vi "Interface_ImplementInterface.vi"(7 "Action":T1=enum."GeneratePattern", 8 "error in (no error)":errorcluster, 10 "DataIn":variant, 11 "ClassRefToActOn":refnum<vi>) -> (0 "error out":errorcluster, 1 "Name":string, 2 "DataOut":variant, 3 "Cancelled":bool)   [LabVIEW 2012]
uses:
  <resource>/Framework/Providers/Open_GDS/ClassProviders/Provider_BaseClassInterface/BaseProvider_SubVIs/BaseProvider_DesignPatternsActions.ctl
  <resource>/Framework/Providers/Open_GDS/ClassProviders/DesignPatterns/Interface/Interface_SubVIs/InterfaceType.ctl
  <resource>/Framework/Providers/Open_GDS/ClassProviders/Common/LvIcon_class/GDSLvIcon_ClassColorTypes.ctl
  <vilib>/picture/picture.llb/imagedata.ctl
  <vilib>/Utility/miscctls.llb/LVPointTypeDef.ctl
  <resource>/Framework/Providers/Open_GDS/ClassProviders/Provider_BaseClassInterface/ClassWriter_class/ClassWriter.lvclass
panel:
  in  "Interfaces":u16(ring) items=["I1-GOOP4.lvclass (By VI Server)", "I1-Native.lvclass (By VI Server)"]
  in  "_Cancel":bool
  in  "_OK":bool
  # "Implement Interface"
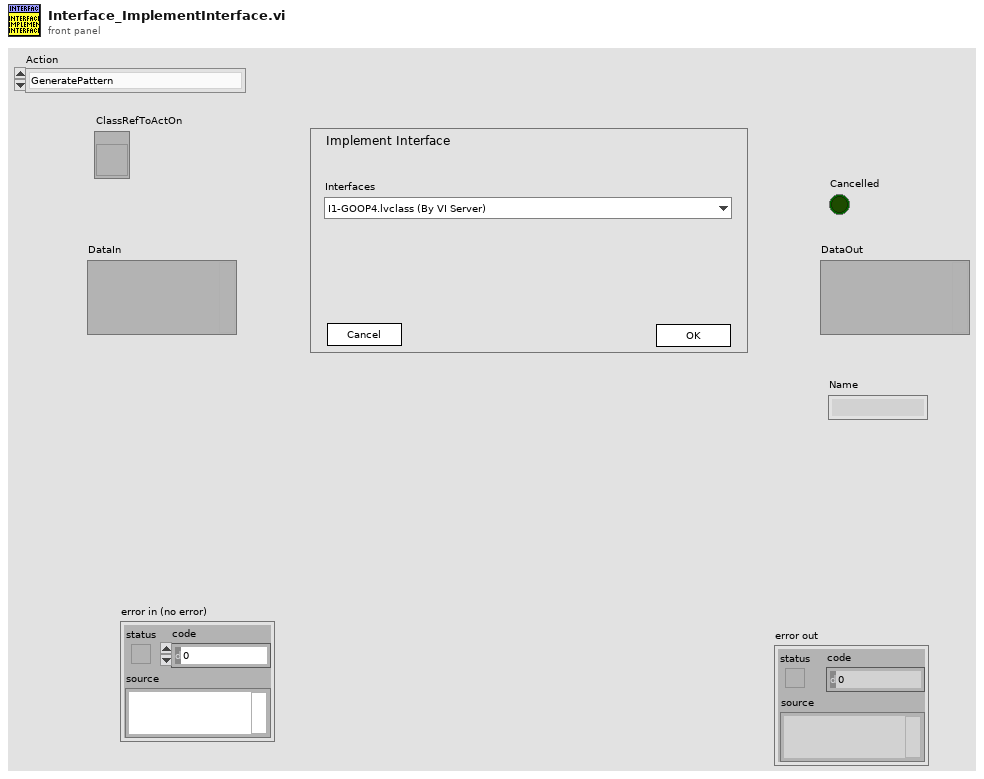
[diagram p1: front panel]
types:
  T1 = typedef "BaseProvider_DesignPatternsActions.ctl" = enum16{"AddPatternDialog", "GeneratePattern", "RemovePattern", "CreatePatternMethod", "UpdatePattern"}
  T2 = typedef "InterfaceType.ctl" = enum16{"ByAggregation", "ByViServer"}
  T3 = cluster{"Application":refnum<vi>, "ClassName":string, "BaseInterfaceClass":path, "ClassFolder":path, "BaseInterfaceClassRef":refnum<vi>, "NewInterfaceClassRef":refnum<vi>, "I_MethodRefs":refnum<vi>[], "C_MethodRefs":refnum<vi>[], "SubViUpperLeftTerminal":refnum<vi>[], "RefNameInSubInterface":string, "GetRefVI":path, "BaseInterfaceName":string, "RefNameInClass":string, "ImplementVI":path, "SubInterfaceImplementVI":path, "GetVIRef":refnum<vi>, "ImplementViRef":refnum<vi>, "SubInterfaceClassName":string, "FullClassName":string, "Type":T2}
  T4 = enum32{"Invalid", "Default", "Floating", "Floating/Auto-Hide", "Modal"}
  T5 = cluster{"Cancelled":bool, "Files":path[], "ClassPath":path, "DataOut":variant, "Interfaces":refnum<vi>[], "Type":T2[]}
  T6 = typedef "GDSLvIcon_ClassColorTypes.ctl" = cluster{"Frame":u32, "Header Text Color":u32, "Header Background":u32, "BodyBackgroundPublic":u32, "BodyBackgroundProtected":u32, "BodyBackgroundPrivate":u32, "Body Text Color":u32, "Frame thickness":u8, "ProtectedPrivateSame":bool, "Icon Header Size":u8, "Font Compression":enum16{"Auto", "On", "Off"}, "CapitalOnly":bool}
  T7 = typedef "imagedata.ctl" = cluster{"image type":i32, "image depth":i32, "image":u8[], "mask":u8[], "colors":u32[], "Rectangle":cluster{"left":i16, "top":i16, "right":i16, "bottom":i16}}
  T8 = enum16{"UINT8", "INT8", "UINT16", "INT16", "UINT32", "INT32", "UINT64", "INT64", "SGL", "DBL", "EXT", "CSG", "CDB", "CXT", "TimeStamp", "STRING", "PATH", "BOOL", "ENUM", "RefNum", "VIRefNum", "ClassRefNum", "Cluster", "Variant", "TypeRef", "Waveform", "LabVIEW Object", "Other"}
  T9 = typedef "LVPointTypeDef.ctl" = cluster{"Horizontal":i16, "Vertical":i16}
  T10 = typedef "GDSLvCLass_ClassSettingsType.ctl" = cluster{"ClassProviderName":string, "ClassTemplateUsed":string, "ClassTemplateVersion":string, "ClassDescription":string, "PlugIns":T11[], "ConnectorPanePattern":string}
  T11 = typedef "GDSLvClass_PlugIn.ctl" = cluster{"Type":T12, "ID":string, "Version":string, "Path":path, "Name":string, "Data":variant}
  T12 = typedef "GDSLvClass_PlugInTypes.ctl" = enum16{"DesignPattern", "MethodTypes"}
  T13 = typedef "GDSLvClass_IconSettingsType.ctl" = cluster{"Frame":u32, "Frame thickness":u8, "Header Background":u32, "Header Text":u32, "ColorPublic":u32, "ColorProtected":u32, "ColorPrivate":u32, "Body Text":u32, "ClassBodyIcon":string}
  T14 = cluster{"Foreground Color":u32, "Background Color":u32, "Fill Pattern":cluster{"Row 0":u8, "Row 1":u8, "Row 2":u8, "Row 3":u8, "Row 4":u8, "Row 5":u8, "Row 6":u8, "Row 7":u8}, "Width":i16, "Mode":enum16{"Copy", "Or", "Exclusive Or", "Bit Clear", "Not Copy", "Not Or", "Nor Exclusive Or", "Not Bit Clear"}, "Style":enum32{"Solid", "Dash", "Dot", "Dash Dot", "Dash Dot Dot"}, "Fill Rule":enum32{"Even Odd", "Winding"}, "End Caps":enum32{"Default", "Flat"}}[]
  T15 = enum16{"UINT8", "INT8", "UINT16", "INT16", "UINT32", "INT32", "UINT64", "INT64", "SGL", "DBL", "EXT", "CSG", "CDB", "CXT", "TimeStamp", "STRING", "PATH", "BOOL", "ENUM", "RefNum", "VIRefNum", "ClassRefNum", "Cluster", "Variant", "TypeRef", "Waveform", "LabVIEW Object", "Other"}[]
  T16 = typedef "LVRectTypeDef.ctl" = cluster{"Left":i16, "Top":i16, "Right":i16, "Bottom":i16}
  T17 = typedef "LVPositionTypeDef.ctl" = cluster{"Left":i32, "Top":i32}
  T18 = cluster{"Alignment":enum32{"Left", "Right", "Hybrid", "Center", "Gravity"}, "Rules":enum32{"Strict", "Allow Wires Under Labels", "Allow Wires Under Lead Nodes", "Allow Wires Under Wide Blocks"}, "Max Heuristic Iterations":u32, "Max Simplex Iterations":u32, "Block Padding":cluster{"Horizontal":i32, "Vertical":i32}, "Wire Padding":cluster{"Horizontal":i32, "Vertical":i32}, "Auto-Tune by Topology":bool, "Fine-Tune Y Positions":bool, "Align All Controls on Left":bool, "Align All Indicators on Right":bool, "Use Array Dimension Heuristics":bool}
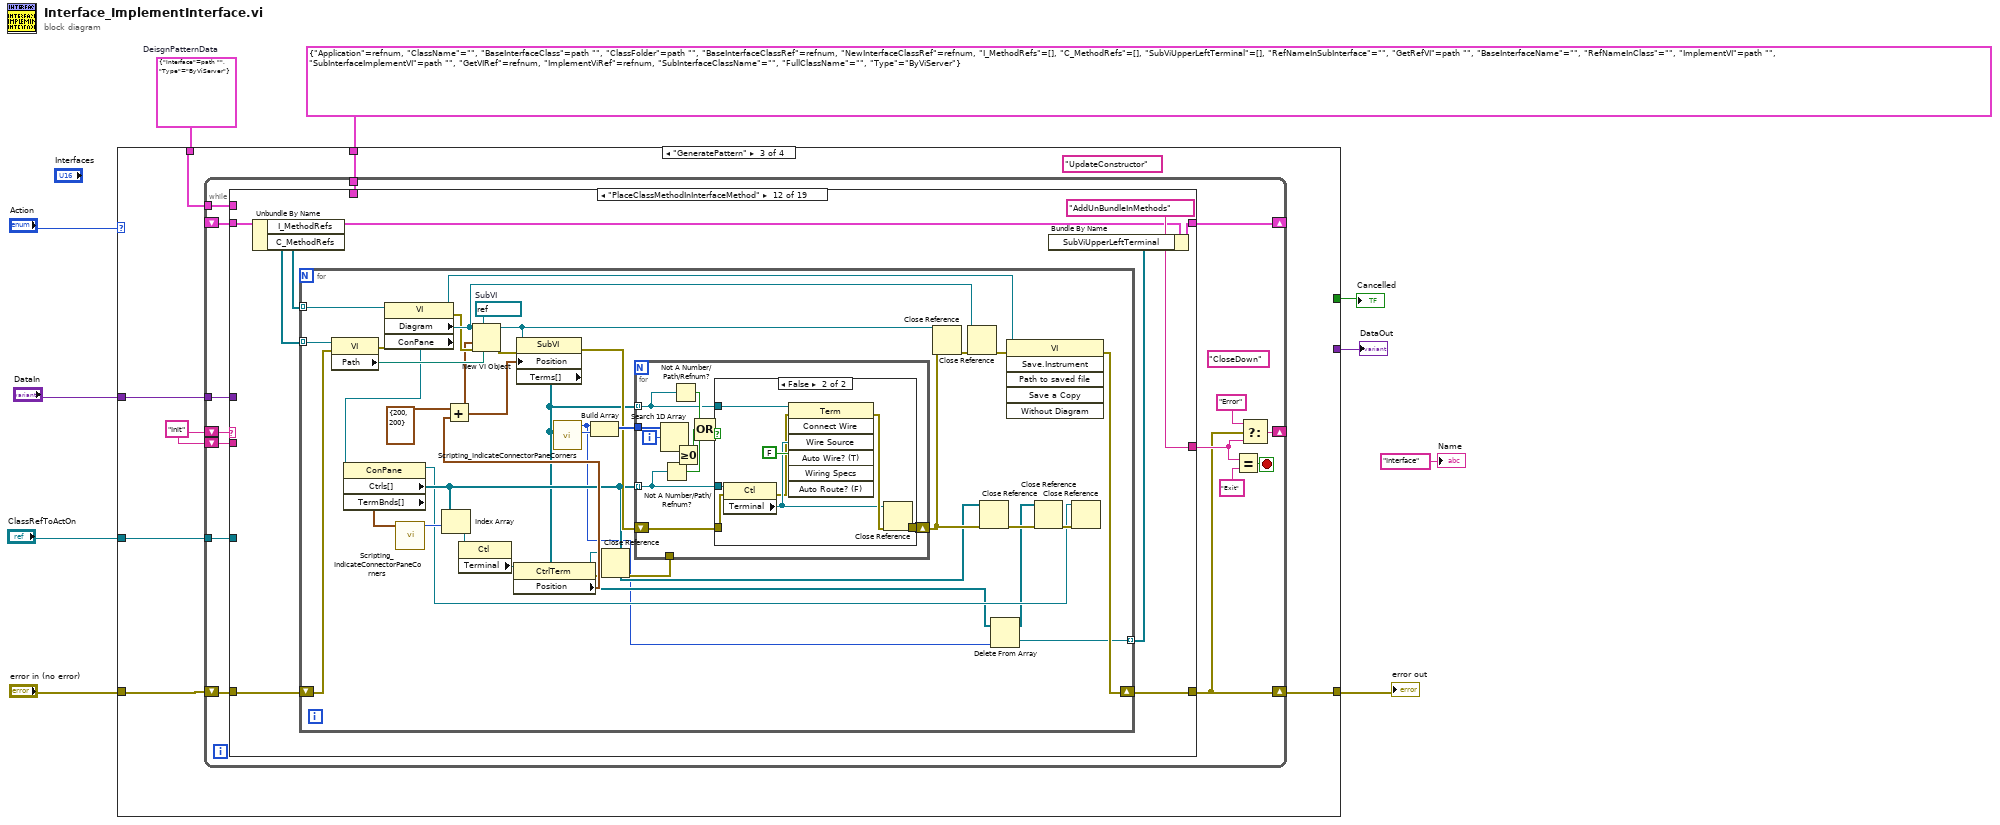
[diagram p0: block diagram]
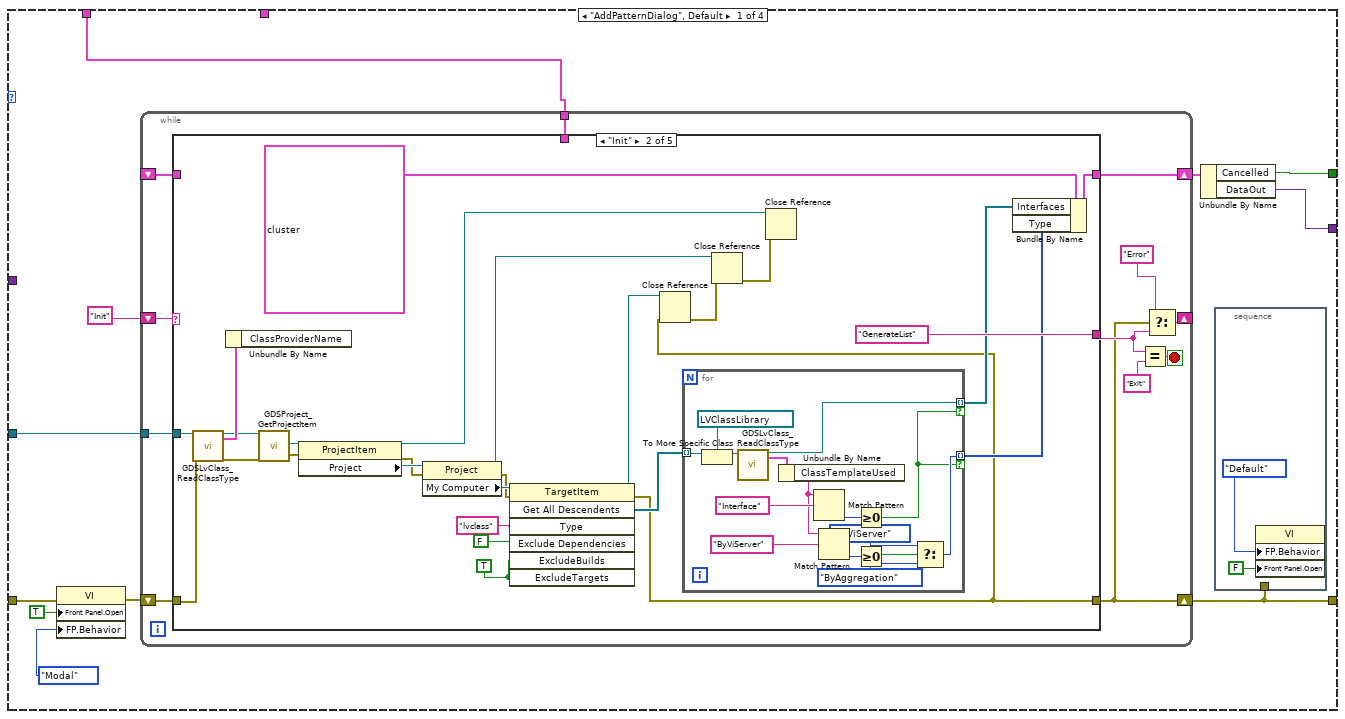
[diagram p2: hidden frame]
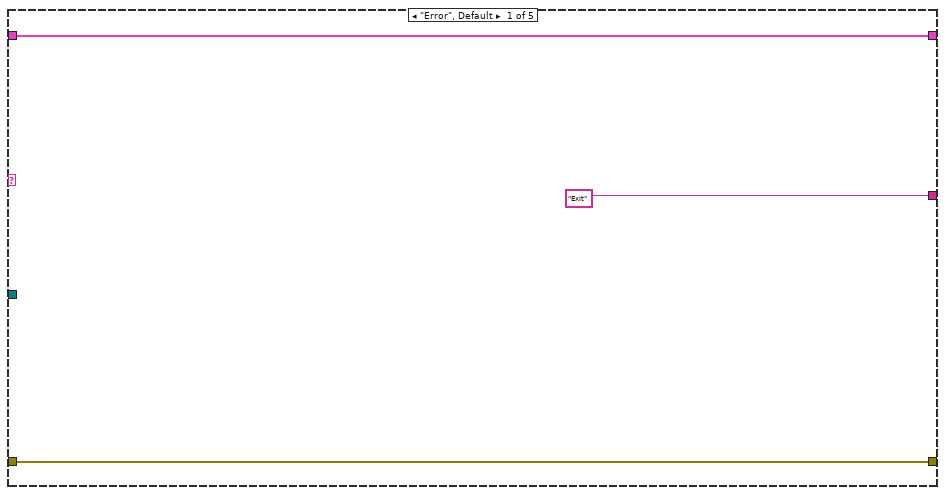
[diagram p3: hidden frame]
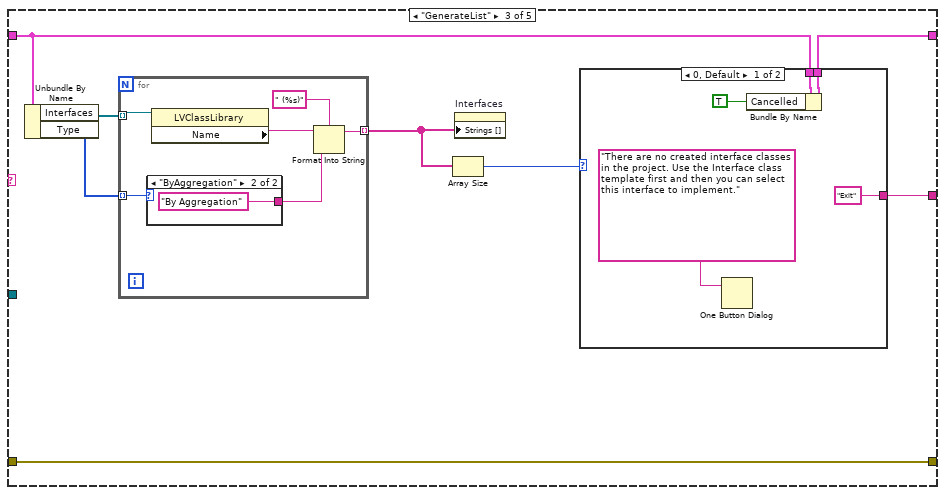
[diagram p4: hidden frame]
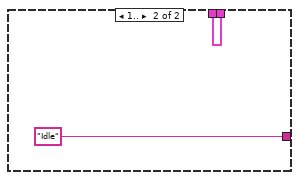
[diagram p5: hidden frame]
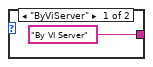
[diagram p6: hidden frame]
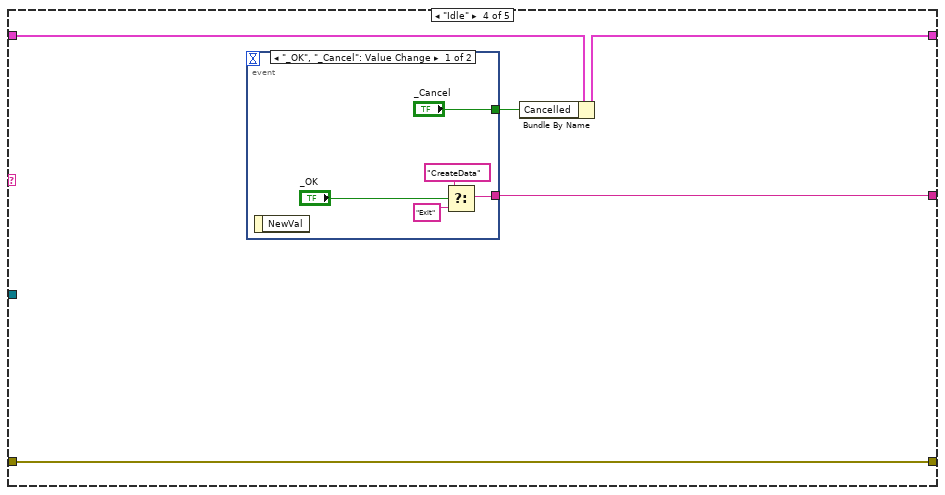
[diagram p7: hidden frame]
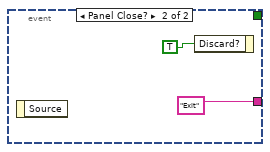
[diagram p8: hidden frame]
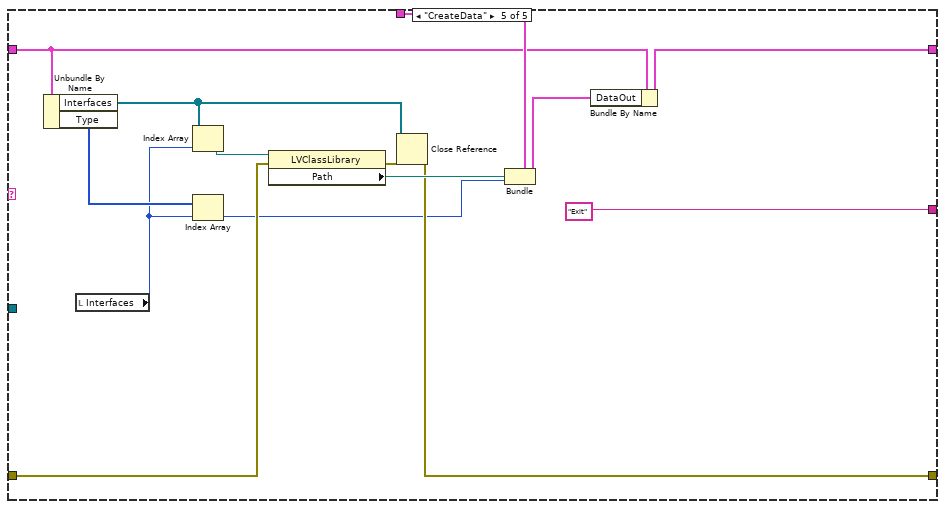
[diagram p9: hidden frame]
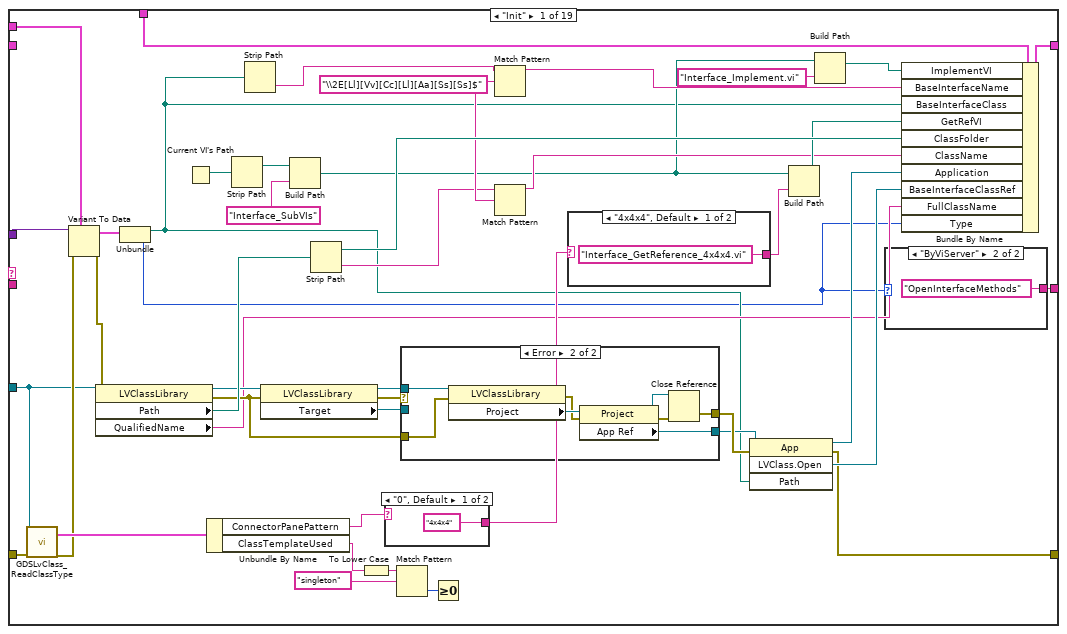
[diagram p11: hidden frame]
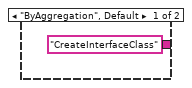
[diagram p12: hidden frame]
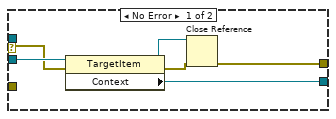
[diagram p13: hidden frame]
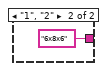
[diagram p14: hidden frame]
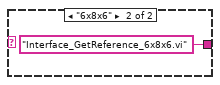
[diagram p15: hidden frame]
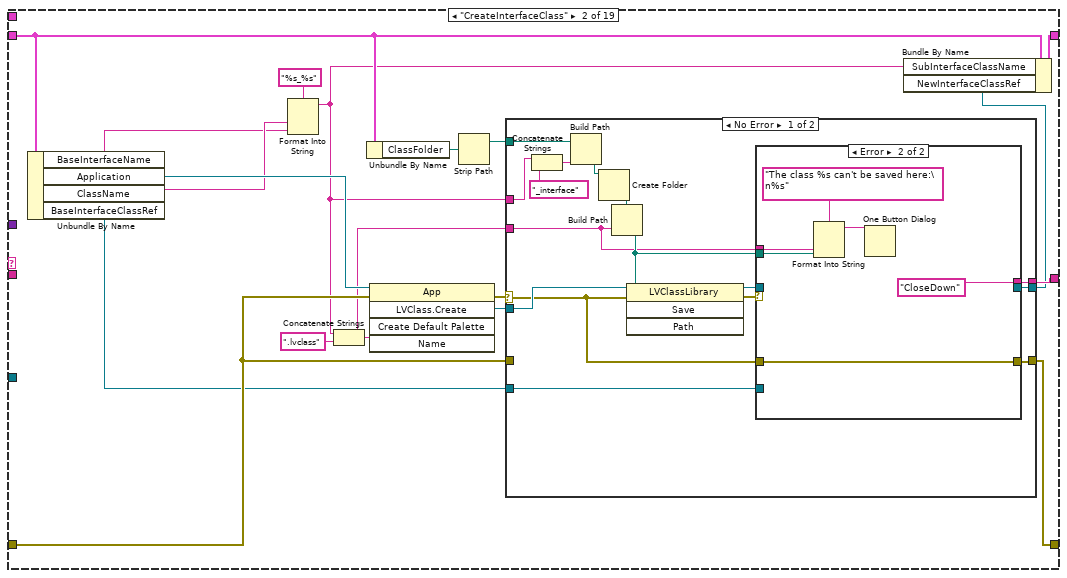
[diagram p16: hidden frame]
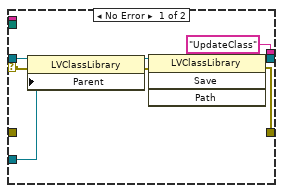
[diagram p17: hidden frame]
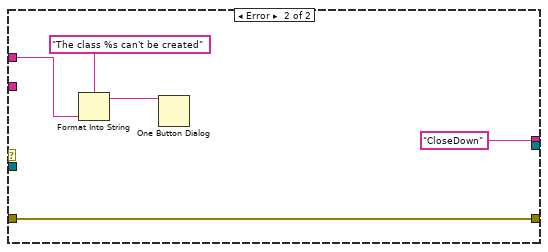
[diagram p18: hidden frame]
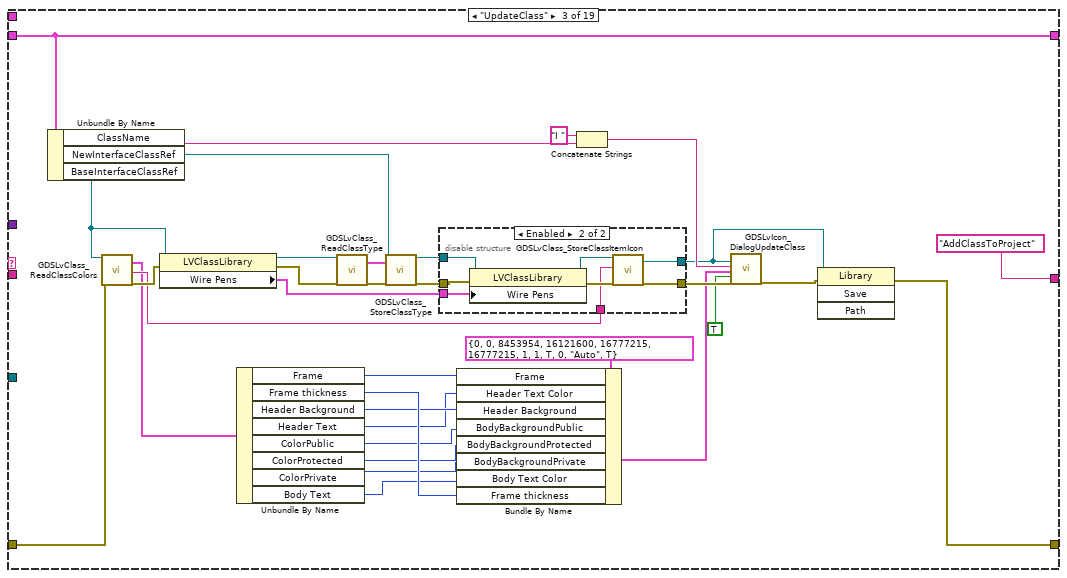
[diagram p19: hidden frame]
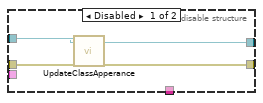
[diagram p20: hidden frame]
diagram:
  w4 = cluster{"Interface":path, "Type":T2} {"Interface"=path "", "Type"=enum."ByViServer"}  # DeisgnPatternData
  n1 = case shown="\"GeneratePattern\"" "Action" {
    tunnel: "error in (no error)" -> [w20 w129 w130 w891]
    tunnel: [w17 w129 w136 w890] -> w8
    tunnel: "ClassRefToActOn" -> [w15 _ w132 _]
    tunnel: [w14 _ _ _] -> w6
    tunnel: [w13 _ _ _] -> w5
    tunnel: w4 -> [w12 _ w134 _]
    tunnel: "DataIn" -> [_ _ w135 _]
    tunnel: T3 {"Application"=refnum, "ClassName"="", "BaseInterfaceClass"=path "", "ClassFolder"=path "", "BaseInterfaceClassRef"=refnum, "NewInterfaceClassRef"=refnum, "I_MethodRefs"=[], "C_MethodRefs"=[], "SubViUpperLeftTerminal"=[], "RefNameInSubInterface"="", "GetRefVI"=path "", "BaseInterfaceName"="", "RefNameInClass"="", "ImplementVI"=path "", "SubInterfaceImplementVI"=path "", "GetVIRef"=refnum, "ImplementViRef"=refnum, "SubInterfaceClassName"="", "FullClassName"="", "Type"=enum."ByViServer"} -> [_ _ w133 _]
    frame "AddPatternDialog", Default {
      n2 = property class="VI"(error in=w20, "Front Panel.Open"=TRUE ("Front Panel Window:Open"), "FP.Behavior"=T4."Modal" ("Front Panel Window:Behavior")) -> (error out=w19:errorcluster)  [unwired: 1 in, 1 out]
      n3 = while {
        shift-right: [w28] -> w17
        shift-left: w19 -> [w35]
        shift-right: [w33] -> _
        shift-left: "Init" -> [w34]
        shift-right: [w27] -> w16
        shift-left: _ -> [w26]
        tunnel: w15 -> [w25]
        tunnel: w12 -> [w24]
        stop <- w32 stop-if-true
        n4 = case shown="\"Init\"" w34 {
          tunnel: w35 -> [w38 w57 w85 w106 w119]
          tunnel: [w38 w39 w85 w106 w118] -> w28
          tunnel: ["Exit" "GenerateList" w86 w107 "Exit"] -> w29
          tunnel: [w36 w59 w81 w105 w127] -> w27
          tunnel: w26 -> [w36 _ w82 w103 w124]
          tunnel: w25 -> [_ w58 _ _ _]
          tunnel: w24 -> [_ _ _ _ w125]
          frame "Error", Default {
          }
          frame "Init" {
            w47 = TRUE ("ExcludeDependencies")
            n5 = call <resource>:"GDSLvClass_ReadClassType.vi"("Class Refnum In"=w58, "error in (no error)"=w57) -> ("Class Refnum Out"=w55:refnum<vi>, "ClassSettings"=w56:T10, "error out"=w54:errorcluster)  [unwired: 15 in]
            n6 = Unbundle By Name(w56) -> ()  [unwired: 1 out]
            n7 = call <resource>:"GDSProject_GetProjectItem.vi"("ProjectItemToSearchFrom"=w55, "error in (no error)"=w54) -> ("ProjectItemFound"=w53:refnum<vi>, "error out"=w52:errorcluster)  [unwired: 14 in, 2 out]
            n8 = property class="ProjectItem"(reference=w53, error in=w52) -> (reference out=w41:refnum<vi>, error out=w48:errorcluster, "Project"=w51:refnum<vi>)
            n9 = property class="Project"(reference=w51, error in=w48) -> (reference out=w43:refnum<vi>, error out=w49:errorcluster, "My Computer"=w50:refnum<vi>)
            n10 = invoke class="TargetItem" method="Get All Descendents"(reference=w50, error in=w49, "Type"="lvclass", "Exclude Dependencies"=FALSE ("ExcludeDependencies"), "ExcludeBuilds"=w47, "ExcludeTargets"=w47) -> (reference out=w45:refnum<vi>, error out=w39:errorcluster, "All Descendents"=w61:refnum<vi>[])  [unwired: 1 in, 4 out]
            n11 = Close Reference(reference=w45, error in (no error)=w39) -> (error out=w44:errorcluster)
            n12 = for {
              tunnel: w61 -> [w79] mode=indexing
              tunnel: [w73] -> w46 mode=indexing if=w65
              tunnel: [w66] -> w40 mode=indexing if=w65
              n13 = To More Specific Class(target class=refnum<vi> refnum ("Class Refnum In"), reference=w79) -> (specific class reference=w77:refnum<vi>)  [unwired: 1 in, 1 out]
              n14 = call <resource>:"GDSLvClass_ReadClassType.vi"("Class Refnum In"=w77) -> ("Class Refnum Out"=w73:refnum<vi>, "ClassSettings"=w76:T10)  [unwired: 16 in, 1 out]
              n15 = Unbundle By Name(w76) -> ("ClassTemplateUsed"=w72:string)
              n16 = Match Pattern(string=w72, regular expression="Interface") -> (offset past match=w74:i32)  [unwired: 1 in, 3 out]
              n17 = Match Pattern(string=w72, regular expression="ByViServer") -> (offset past match=w70:i32)  [unwired: 1 in, 3 out]
              n18 = Greater Or Equal To 0?(x=w74) -> (x >= 0?=w65:bool)
              n19 = Greater Or Equal To 0?(x=w70) -> (x >= 0?=w69:bool)
              n20 = Select(t=InterfaceType."ByViServer" ("Type"), s=w69, f=InterfaceType."ByAggregation" ("Type")) -> (s? t:f=w66:T2)
            }
            n21 = Close Reference(reference=w43, error in (no error)=w44) -> (error out=w42:errorcluster)
            n22 = Close Reference(reference=w41, error in (no error)=w42) -> ()  [unwired: 1 out]
            n23 = Bundle By Name(cluster=T5 {"Cancelled"=FALSE, "Files"=[], "ClassPath"=path "", "DataOut"=variant, "Interfaces"=[], "Type"=[]}, "Interfaces"=w46, "Type"=w40) -> (w59:T5)
          }
          frame "GenerateList" {
            n24 = Unbundle By Name(w82) -> ("Interfaces"=w87:refnum<vi>[], "Type"=w80:T2[])
            n25 = for {
              tunnel: w87 -> [w100] mode=indexing
              tunnel: [w98] -> w84 mode=indexing
              tunnel: w80 -> [w96] mode=indexing
              n26 = case shown="\"ByAggregation\"" w96 {
                tunnel: ["By VI Server" ("format string") "By Aggregation" ("format string")] -> w95
                frame "ByViServer" {
                }
                frame "ByAggregation" {
                }
              }
              n27 = property class="LVClassLibrary"(reference=w100) -> ("Name"=w99:string)  [unwired: 1 in, 2 out]
              n28 = Format Into String(format string=" (%s)", initial string=w99, w95) -> (resulting string=w98:string)  [unwired: 1 in, 1 out]
            }
            n29 = Array Size(array=w84) -> (size(s)=w83:i32)
            n30 = property on="Interfaces" class="Ring (strict)"("Strings []"=w84) -> ()  [unwired: 2 in, 2 out]
            n31 = case shown="0, Default" w83 {
              tunnel: ["Exit" "Idle"] -> w86
              tunnel: w82 -> [w90 w93]
              tunnel: [w89 w93] -> w81
              frame 0, Default {
                n32 = One Button Dialog(message="There are no created interface classes in the project. Use the Interface class template first and then you can select this interface to implement.") -> ()  [unwired: 1 in, 1 out]
                n33 = Bundle By Name(cluster=w90, "Cancelled"=TRUE) -> (w89:T5)
              }
              frame 1.. {
              }
            }
          }
          frame "Idle" {
            n34 = event shown="[0] \"_OK\", \"_Cancel\": Value Change" {
              selector: _ -> [_ _]
              dyn-events: _ -> [_ _]
              timeout: _ -> [_ _]
              tunnel: [w111 "Exit"] -> w107
              tunnel: ["_Cancel" _] -> w104
              event "_OK", "_Cancel": Value Change {
                n35 = event-data() -> ()  [unwired: 1 in, 1 out]
                n36 = Select(t="CreateData", s="_OK", f="Exit") -> (s? t:f=w111:string)
              }
              event Panel Close? {
                n37 = event-data() -> ()  [unwired: 1 in, 1 out]
                n38 = event-data("Discard?"=TRUE) -> ()  [unwired: 1 in, 1 out]
              }
            }
            n39 = Bundle By Name(cluster=w103, "Cancelled"=w104) -> (w105:T5)
          }
          frame "CreateData" {
            n40 = Unbundle By Name(w124) -> ("Interfaces"=w120:refnum<vi>[], "Type"=w117:T2[])
            n41 = local read "Interfaces"() -> (w116:u16)
            n42 = Index Array(array=w120, index=w116) -> (element=w123:refnum<vi>)
            n43 = Index Array(array=w117, index=w116) -> (element=w115:T2)
            n44 = property class="LVClassLibrary"(reference=w123, error in=w119) -> (error out=w121:errorcluster, "Path"=w122:path)  [unwired: 1 out]
            n45 = Close Reference(reference=w120, error in (no error)=w121) -> (error out=w118:errorcluster)
            n46 = Bundle(cluster=w125, "Interface"=w122, "Type"=w115) -> (w128:cluster{"Interface":path, "Type":T2})
            n47 = Bundle By Name(cluster=w124, "DataOut"=w128) -> (w127:T5)
          }
        }
        n48 = Equal?(x=w29, y="Exit") -> (x = y?=w32:bool)
        n49 = Select(t="Error", s=w28, f=w29) -> (s? t:f=w33:string)
      }
      n50 = Unbundle By Name(w16) -> ("Cancelled"=w14:bool, "DataOut"=w13:variant)
      n51 = stacked-sequence {
        tunnel: w17 -> [_]
        frame #0 {
          n52 = property class="VI"("FP.Behavior"=T4."Default" ("Front Panel Window:Behavior"), "Front Panel.Open"=FALSE ("Front Panel Window:Open")) -> ()  [unwired: 2 in, 2 out]
        }
      }
    }
    frame "RemovePattern" {
    }
    frame "GeneratePattern" {
      (unwired) "UpdateConstructor"
      w131 = "Init"
      n53 = while {
        shift-right: [w144] -> w136
        shift-left: w130 -> [w151]
        shift-right: [w149] -> _
        shift-left: w131 -> [w150]
        shift-right: [w143] -> _
        shift-left: _ -> [w142]
        tunnel: w135 -> [w141]
        tunnel: w134 -> [w140]
        tunnel: w133 -> [w139]
        tunnel: w132 -> [w138]
        shift-left: w131 -> [w137]
        stop <- w148 stop-if-true
        (unwired) "CloseDown"
        n54 = case shown="\"PlaceClassMethodInInterfaceMethod\"" w150 {
          tunnel: w151 -> [w173 w230 w289 w324 w330 w397 w420 w433 w464 w497 w537 w545 w613 w691 w751 w791 w852 w856 w864]
          tunnel: [w182 w229 w290 w315 w327 w396 w422 w434 w458 w496 w507 w544 w611 w687 w728 w786 w826 w855 w869] -> w144
          tunnel: [w196 w231 "AddClassToProject" "CreateInterfaceMethods" "UpdateMethods" "CreateNewMethodsInClass" "CleanUpMethods" "CreateNewMethodsInClass" "CopyControlsToClassMethods" w498 "PlaceClassMethodInInterfaceMethod" "AddUnBundleInMethods" "CreateGetRefMethod" "UpdateGetRefIcon" "AddImplementVIInInterfaceSubClass" "UpdateImplementIcon" "UpdateConstructor" "CloseDown" "Exit"] -> w145
          tunnel: [w195 w222 w301 w318 w338 w398 w417 w431 w460 w493 w518 w541 w612 w664 w753 w763 w853 w860 w865] -> w143
          tunnel: w142 -> [_ w223 w301 w318 w340 w400 w417 w431 w461 w493 w519 w542 w612 w665 w753 w764 w853 w860 w865]
          tunnel: w141 -> [w194 _ _ _ _ _ _ _ _ _ _ _ _ _ _ _ _ _ _]
          tunnel: w140 -> [w193 _ _ _ _ _ _ _ _ _ _ _ _ _ _ _ _ _ _]
          tunnel: w139 -> [w192 _ _ _ _ _ _ _ _ _ _ _ _ _ _ _ _ _ _]
          tunnel: w138 -> [w171 _ _ w325 _ _ _ _ w463 _ w538 _ _ w704 w752 w766 _ w854 w871]
          tunnel: w137 -> [_ _ _ _ _ _ _ _ _ _ _ _ _ _ _ _ _ _ w866]
          frame "Init" {
            w167 = "\\2E[Ll][Vv][Cc][Ll][Aa][Ss][Ss]$" ("regular expression")
            n55 = call <resource>:"GDSLvClass_ReadClassType.vi"("Class Refnum In"=w171, "error in (no error)"=w173) -> ("ClassSettings"=w179:T10, "error out"=w172:errorcluster)  [unwired: 15 in, 1 out]
            n56 = Variant To Data(error in=w172, type=w193, Variant=w194) -> (data=w186:cluster{"Interface":path, "Type":T2}, error out=w188:errorcluster)
            n57 = property class="LVClassLibrary"(reference=w171, error in=w188) -> (reference out=w158:refnum<vi>, error out=w157:errorcluster, "Path"=w187:path, "QualifiedName"=w154:string)
            n58 = Unbundle(w186) -> ("Interface"=w153:path, "Type"=w152:T2)
            n59 = Current VI's Path() -> (path=w191:path)
            n60 = Unbundle By Name(w179) -> ("ConnectorPanePattern"=w178:string, "ClassTemplateUsed"=w177:string)
            n61 = Strip Path(path=w191) -> (stripped path=w190:path)  [unwired: 1 out]
            n62 = Strip Path(path=w153) -> (name=w169:string)  [unwired: 1 out]
            n63 = property class="LVClassLibrary"(reference=w158, error in=w157) -> (reference out=w161:refnum<vi>, error out=w159:errorcluster, "Target"=w160:refnum<vi>)
            n64 = Build Path(base path=w190, name or relative path="Interface_SubVIs") -> (appended path=w164:path)
            n65 = Strip Path(path=w187) -> (stripped path=w185:path, name=w166:string)
            n66 = To Lower Case(string=w177) -> (all lower case string=w175:string)
            n67 = case shown="\"0\", Default" w178 {
              tunnel: ["4x4x4" "6x8x6"] -> w170
              frame "0", Default {
              }
              frame "1", "2" {
              }
            }
            n68 = Match Pattern(string=w175, regular expression="singleton" ("search string")) -> (offset past match=w176:i32)  [unwired: 1 in, 3 out]
            n69 = case shown="Error" w159 {
              selector: w159 -> [w200 _]
              tunnel: w160 -> [w204 _]
              tunnel: [w203 w206] -> w155
              tunnel: [w199 w207] -> w156
              tunnel: w161 -> [_ w212]
              tunnel: w157 -> [_ w211]
              frame No Error {
                n70 = property class="TargetItem"(reference=w204, error in=w200) -> (reference out=w201:refnum<vi>, error out=w202:errorcluster, "Context"=w203:refnum<vi>)
                n71 = Close Reference(reference=w201, error in (no error)=w202) -> (error out=w199:errorcluster)
              }
              frame Error {
                n72 = property class="LVClassLibrary"(reference=w212, error in=w211) -> (error out=w205:errorcluster, "Project"=w210:refnum<vi>)  [unwired: 1 out]
                n73 = property class="Project"(reference=w210, error in=w205) -> (reference out=w208:refnum<vi>, error out=w209:errorcluster, "App Ref"=w206:refnum<vi>)
                n74 = Close Reference(reference=w208, error in (no error)=w209) -> (error out=w207:errorcluster)
              }
            }
            n75 = Greater Or Equal To 0?(x=w176) -> ()  [unwired: 1 out]
            n76 = Match Pattern(string=w169, regular expression=w167) -> (before substring=w168:string)  [unwired: 1 in, 3 out]
            n77 = Match Pattern(string=w166, regular expression=w167) -> (before substring=w165:string)  [unwired: 1 in, 3 out]
            n78 = case shown="\"4x4x4\", Default" w170 {
              tunnel: ["Interface_GetReference_4x4x4.vi" ("name or relative path") "Interface_GetReference_6x8x6.vi" ("name or relative path")] -> w181
              frame "4x4x4", Default {
              }
              frame "6x8x6" {
              }
            }
            n79 = invoke class="App" method="LVClass.Open"(reference=w155, error in=w156, "Path"=w153) -> (reference out=w184:refnum<vi>, error out=w182:errorcluster, "LVClass.Open"=w183:refnum<vi>)  [unwired: 1 in, 1 out]
            n80 = Build Path(base path=w164, name or relative path=w181) -> (appended path=w180:path)
            n81 = Build Path(base path=w164, name or relative path="Interface_Implement.vi") -> (appended path=w162:path)
            n82 = case shown="\"ByViServer\"" w152 {
              tunnel: ["CreateInterfaceClass" "OpenInterfaceMethods"] -> w196
              frame "ByAggregation", Default {
              }
              frame "ByViServer" {
              }
            }
            n83 = Bundle By Name(cluster=w192, "ImplementVI"=w162, "BaseInterfaceName"=w168, "BaseInterfaceClass"=w153, "GetRefVI"=w180, "ClassFolder"=w185, "ClassName"=w165, "Application"=w184, "BaseInterfaceClassRef"=w183, "FullClassName"=w154, "Type"=w152) -> (w195:T3)
          }
          frame "CreateInterfaceClass" {
            n84 = Unbundle By Name(w223) -> ("BaseInterfaceName"=w218:string, "Application"=w234:refnum<vi>, "ClassName"=w219:string, "BaseInterfaceClassRef"=w224:refnum<vi>)
            n85 = Format Into String(format string="%s_%s", w219, w218) -> (resulting string=w217:string)  [unwired: 2 in, 1 out]
            n86 = Concatenate Strings(w217, ".lvclass" ("string")) -> (w220:string)
            n87 = Unbundle By Name(w223) -> ("ClassFolder"=w227:path)
            n88 = invoke class="App" method="LVClass.Create"(reference=w234, error in=w230, "Name"=w220) -> (error out=w232:errorcluster, "LVClass.Create"=w228:refnum<vi>)  [unwired: 2 in, 3 out]
            n89 = Strip Path(path=w227) -> (stripped path=w226:path)  [unwired: 1 out]
            n90 = case shown="No Error" w232 {
              selector: w232 -> [w243 _]
              tunnel: w217 -> [w236 w269]
              tunnel: [w244 "CloseDown"] -> w231
              tunnel: w230 -> [_ w265]
              tunnel: [w242 w265] -> w229
              tunnel: w228 -> [w250 _]
              tunnel: w226 -> [w249 _]
              tunnel: w224 -> [w240 _]
              tunnel: [w239 _] -> w221
              tunnel: w220 -> [w235 _]
              frame No Error {
                n91 = Concatenate Strings(w236, "_interface" ("format string")) -> (w247:string)
                n92 = Build Path(base path=w249, name or relative path=w247) -> (appended path=w238:path)
                n93 = Create Folder(path (use dialog)=w238) -> (created path=w237:path)  [unwired: 2 in, 2 out]
                n94 = Build Path(base path=w237, name or relative path=w235) -> (appended path=w245:path)
                n95 = invoke class="LVClassLibrary" method="Save"(reference=w250, error in=w243, "Path"=w245) -> (reference out=w241:refnum<vi>, error out=w246:errorcluster)  [unwired: 1 in, 2 out]
                n96 = case shown="Error" w246 {
                  selector: w246 -> [w257 _]
                  tunnel: w235 -> [_ w262]
                  tunnel: w245 -> [_ w261]
                  tunnel: ["UpdateClass" "CloseDown"] -> w244
                  tunnel: w243 -> [_ w259]
                  tunnel: [w253 w259] -> w242
                  tunnel: w241 -> [w258 _]
                  tunnel: w240 -> [w256 _]
                  tunnel: [w252 _] -> w239
                  frame No Error {
                    n97 = property class="LVClassLibrary"(reference=w258, error in=w257, "Parent"=w256) -> (reference out=w255:refnum<vi>, error out=w254:errorcluster)
                    n98 = invoke class="LVClassLibrary" method="Save"(reference=w255, error in=w254) -> (reference out=w252:refnum<vi>, error out=w253:errorcluster)  [unwired: 2 in, 2 out]
                  }
                  frame Error {
                    n99 = Format Into String(format string="The class %s can't be saved here:\n%s" ("message"), w262, w261) -> (resulting string=w263:string)  [unwired: 2 in, 1 out]
                    n100 = One Button Dialog(message=w263) -> ()  [unwired: 1 in, 1 out]
                  }
                }
              }
              frame Error {
                n101 = Format Into String(format string="The class %s can't be created" ("message"), w269) -> (resulting string=w267:string)  [unwired: 2 in, 1 out]
                n102 = One Button Dialog(message=w267) -> ()  [unwired: 1 in, 1 out]
              }
            }
            n103 = Bundle By Name(cluster=w223, "SubInterfaceClassName"=w217, "NewInterfaceClassRef"=w221) -> (w222:T3)
          }
          frame "UpdateClass" {
            n104 = Unbundle By Name(w301) -> ("ClassName"=w272:string, "NewInterfaceClassRef"=w295:refnum<vi>, "BaseInterfaceClassRef"=w270:refnum<vi>)
            n105 = call <resource>:"GDSLvClass_ReadClassColors.vi"("Library Refnum"=w270, "error in (no error)"=w289) -> ("LvClassIconSettings"=w281:T13, "ClassItemIconName(NoExtension)"=w284:string, "error out"=w287:errorcluster)  [unwired: 12 in, 3 out]
            n106 = property class="LVClassLibrary"(reference=w270, error in=w287) -> (reference out=w288:refnum<vi>, error out=w286:errorcluster, "Wire Pens"=w285:T14)
            n107 = Unbundle By Name(w281) -> ("Frame"=w280:u32, "Frame thickness"=w279:u8, "Header Background"=w278:u32, "Header Text"=w277:u32, "ColorPublic"=w276:u32, "ColorProtected"=w275:u32, "ColorPrivate"=w274:u32, "Body Text"=w273:u32)
            n108 = call <resource>:"GDSLvClass_ReadClassType.vi"("Class Refnum In"=w288, "error in (no error)"=w286) -> ("ClassSettings"=w300:T10, "error out"=w299:errorcluster)  [unwired: 15 in, 1 out]
            n109 = call <resource>:"GDSLvClass_StoreClassType.vi"("Class Refnum In"=w295, "ClassSettings"=w300, "error in (no error)"=w299) -> ("Class Refnum Out"=w298:refnum<vi>, "error out"=w297:errorcluster)  [unwired: 15 in]
            n110 = disable-structure shown="Enabled" {
              disable-tunnel: w298 -> [w306 w313]
              disable-tunnel: w297 -> [w305 w314]
              disable-tunnel: [w304 w308] -> w296
              disable-tunnel: [w303 w307] -> w292
              disable-tunnel: w285 -> [_ w310]
              disable-tunnel: w284 -> [_ w309]
              frame Disabled {
                n111 = call <resource>:"UpdateClassApperance.vi"("ClassRefIn"=w306, "error in (no error)"=w305) -> ("ClassRefOut"=w303:refnum<vi>, "error out"=w304:errorcluster)  [unwired: 16 in]
              }
              frame Enabled {
                n112 = property class="LVClassLibrary"(reference=w313, error in=w314, "Wire Pens"=w310) -> (reference out=w312:refnum<vi>, error out=w311:errorcluster)
                n113 = call <resource>:"GDSLvClass_StoreClassItemIcon.vi"("Library Refnum"=w312, "ClassItemIconName"=w309, "error in (no error)"=w311) -> ("Library Refnum"=w307:refnum<vi>, "error out"=w308:errorcluster)  [unwired: 15 in]
              }
            }
            n114 = Bundle By Name(cluster=T6 {"Frame"=0, "Header Text Color"=0, "Header Background"=8453954, "BodyBackgroundPublic"=16121600, "BodyBackgroundProtected"=16777215, "BodyBackgroundPrivate"=16777215, "Body Text Color"=1, "Frame thickness"=1, "ProtectedPrivateSame"=TRUE, "Icon Header Size"=0, "Font Compression"=enum."Auto", "CapitalOnly"=TRUE} ("Colors"), "Frame"=w280, "Header Text Color"=w277, "Header Background"=w278, "BodyBackgroundPublic"=w276, "BodyBackgroundProtected"=w275, "BodyBackgroundPrivate"=w274, "Body Text Color"=w273, "Frame thickness"=w279) -> (w282:T6)
            n115 = Concatenate Strings("I " ("string"), w272) -> (w293:string)
            n116 = call <resource>:"GDSLvIcon_DialogUpdateClass.vi"("ClassPath(FilePath/ProjectTreePath/LvCLassRef)"=w292, "ClassName"=w293, "Colors"=w282, "AutoUpdate"=TRUE, "error in (no error)"=w296) -> ("error out"=w291:errorcluster)  [unwired: 14 in]
            n117 = invoke class="Library" method="Save"(reference=w292, error in=w291) -> (error out=w290:errorcluster)  [unwired: 2 in, 3 out]
          }
          frame "AddClassToProject" {
            n118 = Unbundle By Name(w318) -> ("NewInterfaceClassRef"=w321:refnum<vi>)
            n119 = property class="LVClassLibrary"(reference=w325, error in=w324) -> (error out=w322:errorcluster, "Parent"=w323:refnum<vi>)  [unwired: 1 out]
            n120 = property class="LVClassLibrary"(reference=w321) -> ("Path"=w320:path)  [unwired: 1 in, 2 out]
            n121 = invoke class="ProjectItem" method="AddFile"(reference=w323, error in=w322, "Path"=w320) -> (reference out=w317:refnum<vi>, error out=w316:errorcluster)  [unwired: 1 in, 2 out]
            n122 = call <resource>:"CommonVIs_Wait.vi"("error in"=w316) -> ("error out"=w315:errorcluster)  [unwired: 9 in]
            n123 = Close Reference(reference=w317, error in (no error)=w315) -> ()  [unwired: 1 out]
          }
          frame "CreateInterfaceMethods" {
            w345 = TRUE ("ExcludeDependencies")
            n124 = Unbundle By Name(w340) -> ("BaseInterfaceClassRef"=w347:refnum<vi>)
            n125 = Unbundle By Name(w340) -> ("NewInterfaceClassRef"=w336:refnum<vi>)
            n126 = invoke class="LVClassLibrary" method="Get All Descendents"(reference=w347, error in=w330, "Type"="VI", "Exclude Dependencies"=w345, "ExcludeBuilds"=w345, "ExcludeTargets"=w345) -> (error out=w343:errorcluster, "All Descendents"=w341:refnum<vi>[])  [unwired: 1 in, 5 out]
            n127 = property class="LVClassLibrary"(reference=w336) -> ("Path"=w335:path, "Member Data"=w326:refnum<vi>)  [unwired: 1 in, 2 out]
            n128 = Not A Number/Path/Refnum?(number/path/refnum=w326) -> (NaN/Path/Refnum?=w331:bool)
            n129 = call <resource>:"GDSLvIcon_AnalyseViIcon.vi"("ViRef/LvCLassRef/LvLibRef/ViPath"=w326) -> ("BodyTextColor"=w329:u32, "FrameColor"=w333:u32, "FrameThickness(1)"=w332:u32, "HeaderIcon"=w334:u8[][], "BodyBkColor"=w328:u32)  [unwired: 6 in, 8 out]
            n130 = Strip Path(path=w335) -> (stripped path=w344:path)  [unwired: 1 out]
            n131 = for {
              tunnel: w341 -> [w372] mode=indexing
              tunnel: w344 -> [w368]
              shift-right: [w361] -> w342
              shift-left: w343 -> [w366]
              tunnel: w336 -> [w364]
              tunnel: [w357] -> w339 mode=indexing
              tunnel: w329 -> [w356]
              tunnel: w334 -> [w355]
              tunnel: w333 -> [w354]
              tunnel: w332 -> [w353]
              tunnel: w331 -> [w351]
              tunnel: w328 -> [w350]
              n132 = property class="ProjectItem"(reference=w372, error in=w366) -> (error out=w365:errorcluster, "Reference"=w371:refnum<vi>, "Path"=w369:path)  [unwired: 1 out]
              n133 = Strip Path(path=w369) -> (name=w367:string)  [unwired: 1 out]
              n134 = Build Path(base path=w368, name or relative path=w367) -> (appended path=w363:path)
              n135 = invoke class="VI" method="Save.Instrument"(reference=w371, error in=w365, "Path to saved file"=w363, "Save a Copy"=TRUE) -> (reference out=w359:refnum<vi>, error out=w360:errorcluster)  [unwired: 2 in, 4 out]
              n136 = Close Reference(reference=w359, error in (no error)=w360) -> ()  [unwired: 1 out]
              n137 = invoke class="LVClassLibrary" method="AddFile"(reference=w364, error in=w360, "Path"=w363) -> (error out=w349:errorcluster, "AddFile"=w362:refnum<vi>)  [unwired: 1 in, 2 out]
              n138 = call <resource>:"CommonVIs_Wait.vi"("error in"=w349) -> ("error out"=w348:errorcluster)  [unwired: 9 in]
              n139 = property class="ProjectItem"(reference=w362, error in=w348) -> (reference out=w358:refnum<vi>, error out=w352:errorcluster, "Reference"=w357:refnum<vi>)
              n140 = case shown="False" w351 {
                tunnel: [w381 w394] -> w361
                tunnel: w357 -> [w380 _]
                tunnel: w356 -> [_ _]
                tunnel: w355 -> [w379 _]
                tunnel: w354 -> [w378 _]
                tunnel: w353 -> [w377 _]
                tunnel: w352 -> [w375 w394]
                tunnel: w350 -> [w374 _]
                frame False {
                  # "Take header from New Class Liberary\nBody Body from current VI\nReplace CurrentBody color with New\nClass Library Body color"
                  n141 = call <resource>:"GDSLvIcon_AnalyseViIcon.vi"("ViRef/LvCLassRef/LvLibRef/ViPath"=w380, "error in (no error)"=w375) -> ("BodyIcon"=w382:u8[][], "BodyBkColor"=w373:u32, "error out"=w376:errorcluster)  [unwired: 5 in, 10 out]
                  n142 = call <resource>:"GDSLvIcon_ReplaceIconColor.vi"("IconIn"=w382, "OldColor"=w373, "NewColor"=w374, "error in (no error)"=w376) -> ("IconOut"=w390:u8[][], "error out"=w388:errorcluster)  [unwired: 14 in]
                  n143 = call <resource>:"GDSLvIcon_CreateIconPicture.vi"("FrameColor"=w378, "FrameThickness(1)"=w377, "HeaderIconIn"=w379, "BodyIconIn"=w390, "error in (no error)"=w388) -> ("WholeIconOut"=w385:u8[][], "error out"=w389:errorcluster)  [unwired: 9 in, 4 out]
                  n144 = Reshape Array(w385, 1024 ("dimension size")) -> (w387:u8[])
                  n145 = Bundle By Name(cluster=T7 {"image type"=0, "image depth"=8, "image"=[], "mask"=[], "colors"=[], "Rectangle"={"left"=0, "top"=0, "right"=32, "bottom"=32}} ("image data"), "image"=w387) -> (w384:T7)
                  n146 = invoke class="VI" method="VI Icon.Set from Image Data"(reference=w380, error in=w389, "ImageData"=w384) -> (reference out=w392:refnum<vi>, error out=w391:errorcluster)  [unwired: 3 in, 4 out]
                  n147 = call <resource>:"Scripting_SaveVi.vi"("ForceResaving(False)"=TRUE, "error in (no error)"=w391, "VIRefToSaveIn"=w392) -> ("error out"=w381:errorcluster)  [unwired: 7 in, 1 out]
                }
                frame True {
                }
              }
              n148 = Close Reference(reference=w358) -> ()  [unwired: 1 in, 1 out]
            }
            n149 = Close Reference(reference=w341, error in (no error)=w342) -> (error out=w327:errorcluster)
            n150 = Bundle By Name(cluster=w340, "I_MethodRefs"=w339) -> (w338:T3)
            n151 = Close Reference(reference=w326, error in (no error)=w327) -> ()  [unwired: 1 out]
          }
          frame "OpenInterfaceMethods" {
            w404 = TRUE ("ExcludeDependencies")
            n152 = Unbundle By Name(w400) -> ("BaseInterfaceClassRef"=w406:refnum<vi>)
            n153 = invoke class="LVClassLibrary" method="Get All Descendents"(reference=w406, error in=w397, "Type"="VI", "Exclude Dependencies"=w404, "ExcludeBuilds"=w404, "ExcludeTargets"=w404) -> (error out=w403:errorcluster, "All Descendents"=w401:refnum<vi>[])  [unwired: 1 in, 5 out]
            n154 = for {
              tunnel: w401 -> [w410] mode=indexing
              shift-right: [w408] -> w402
              shift-left: w403 -> [w409]
              tunnel: [w407] -> w399 mode=indexing
              n155 = property class="ProjectItem"(reference=w410, error in=w409) -> (error out=w408:errorcluster, "Reference"=w407:refnum<vi>)  [unwired: 1 out]
            }
            n156 = Close Reference(reference=w401, error in (no error)=w402) -> (error out=w396:errorcluster)
            n157 = Bundle By Name(cluster=w400, "I_MethodRefs"=w399) -> (w398:T3)
          }
          frame "UpdateMethods" {
            n158 = Unbundle By Name(w417) -> ("I_MethodRefs"=w418:refnum<vi>[])
            n159 = Unbundle By Name(w417) -> ("BaseInterfaceClassRef"=w414:refnum<vi>)
            n160 = Unbundle By Name(w417) -> ("NewInterfaceClassRef"=w421:refnum<vi>)
            n161 = property class="LVClassLibrary"(reference=w421) -> ("Path"=w419:path)  [unwired: 1 in, 2 out]
            n162 = property class="LVClassLibrary"(reference=w414) -> ("Member Data"=w415:refnum<vi>)  [unwired: 1 in, 2 out]
            n163 = property class="VI"(reference=w415) -> (reference out=w411:refnum<vi>, error out=w412:errorcluster, "Path"=w413:path)  [unwired: 1 in]
            n164 = Close Reference(reference=w411, error in (no error)=w412) -> ()  [unwired: 1 out]
            n165 = for {
              tunnel: w413 -> [w426]
              tunnel: w419 -> [w425]
              shift-right: [w423] -> w422
              shift-left: w420 -> [w427]
              tunnel: w418 -> [w424] mode=indexing
              n166 = Build Array(w426) -> (w429:path[])
              n167 = Build Array(w425) -> (w428:path[])
              n168 = call <resource>:"Scripting_ReplaceVisAndControls.vi"("ViRef"=w424, "OldVIsAndControls"=w429, "NewVIsAndControls"=w428, "error in (no error)"=w427) -> ("error out"=w423:errorcluster)  [unwired: 14 in, 1 out]
            }
          }
          frame "CleanUpMethods" {
            n169 = Unbundle By Name(w431) -> ("I_MethodRefs"=w432:refnum<vi>[])
            n170 = for {
              shift-right: [w438] -> w434
              shift-left: w433 -> [w445]
              tunnel: w432 -> [w443] mode=indexing
              n171 = call <resource>:"Scripting_CleanUpControls.vi"("error in (no error)"=w445, "VI-Path/VI-Ref"=w443) -> ("error out"=w444:errorcluster, "ViRef"=w440:refnum<vi>)  [unwired: 8 in]
              n172 = call <resource>:"Scripting_FindNodeOnDiagram.vi"("ViRef(Ignored If Not Wired)"=w440, "NodeTypesToSearchFor"=string[] ["CaseStructure"], "error in (no error)"=w444) -> ("Nodes"=w436:refnum<vi>[], "error out"=w441:errorcluster)  [unwired: 15 in]
              n173 = Empty Array?(array=w436) -> (empty?=w435:bool)
              n174 = case shown="False" w435 {
                tunnel: w441 -> [w451 w454]
                tunnel: w440 -> [w449 w453]
                tunnel: [w448 w454] -> w439
                tunnel: [w447 w453] -> w437
                tunnel: w436 -> [w446 _]
                frame False {
                  n175 = Index Array(array=w446) -> (element=w452:refnum<vi>)  [unwired: 1 in]
                  n176 = invoke class="Node" method="Delete"(reference=w452, error in=w451) -> (error out=w450:errorcluster)  [unwired: 1 in, 2 out]
                  n177 = invoke class="VI" method="BD.Remove Bad Wires"(reference=w449, error in=w450) -> (reference out=w447:refnum<vi>, error out=w448:errorcluster)  [unwired: 1 in, 1 out]
                }
                frame True {
                }
              }
              n178 = invoke class="VI" method="Save.Instrument"(reference=w437, error in=w439) -> (error out=w438:errorcluster)  [unwired: 4 in, 5 out]
              n179 = Close Reference(reference=w436, error in (no error)=w438) -> ()  [unwired: 1 out]
            }
          }
          frame "CreateNewMethodsInClass" {
            n180 = Unbundle By Name(w461) -> ("Application"=w462:refnum<vi>, "I_MethodRefs"=w456:refnum<vi>[])
            n181 = Array Size(array=w456) -> (size(s)=w455:i32)
            n182 = case shown="1.." w455 {
              tunnel: w464 -> [w465 w479]
              tunnel: w463 -> [_ w475]
              tunnel: w462 -> [_ w472]
              tunnel: [_ w471] -> w459
              tunnel: [w465 w469] -> w458
              tunnel: w456 -> [_ w466]
              frame 0, Default {
              }
              frame 1.. {
                n183 = for {
                  tunnel: w466 -> [w491] mode=indexing
                  tunnel: [w488] -> w477 mode=indexing
                  tunnel: [w487] -> w474 mode=indexing
                  n184 = property class="VI"(reference=w491) -> ("Path"=w490:path)  [unwired: 1 in, 2 out]
                  n185 = Strip Path(path=w490) -> (name=w487:string)  [unwired: 1 out]
                  n186 = Match Pattern(string=w487, regular expression=".vi$") -> (before substring=w488:string)  [unwired: 1 in, 3 out]
                }
                n187 = call <resource>:"ReversedEngineering UpdateClassMethods.vi"("ClassPath/LvClassRef"=w475, "Methods"=w477, "error in (no error)"=w479, "Don'tShowDialog(False)"=FALSE, "UseVirtualMethods(True)"=TRUE) -> ("error out"=w470:errorcluster)  [unwired: 14 in]
                n188 = property class="LVClassLibrary"(reference=w475, error in=w470) -> (error out=w473:errorcluster, "Path"=w468:path)  [unwired: 1 out]
                n189 = Strip Path(path=w468) -> (stripped path=w467:path)  [unwired: 1 out]
                n190 = for {
                  tunnel: w474 -> [w486] mode=indexing
                  tunnel: w467 -> [w485]
                  shift-right: [w481] -> w469
                  shift-left: w473 -> [w483]
                  tunnel: w472 -> [w482]
                  tunnel: [w480] -> w471 mode=indexing
                  n191 = Build Path(base path=w485, name or relative path=w486) -> (appended path=w484:path)
                  n192 = Open VI Reference(application reference (local)=w482, vi path=w484, error in (no error)=w483) -> (vi reference=w480:refnum<vi>, error out=w481:errorcluster)  [unwired: 3 in]
                }
              }
            }
            n193 = Bundle By Name(cluster=w461, "C_MethodRefs"=w459) -> (w460:T3)
          }
          frame "CopyControlsToClassMethods" {
            n194 = Unbundle By Name(w493) -> ("C_MethodRefs"=w495:refnum<vi>[], "I_MethodRefs"=w494:refnum<vi>[])
            n195 = for {
              tunnel: w495 -> [w503] mode=indexing
              tunnel: w494 -> [w504] mode=indexing
              shift-right: [w501] -> w496
              shift-left: w497 -> [w505]
              n196 = call <resource>:"Scripting_CopyControlsFromTemplate.vi"("ViRef"=w503, "TemplateVI(Path or Ref)"=w504, "error in (no error)"=w505) -> ("error out"=w502:errorcluster)  [unwired: 16 in]
              n197 = call <resource>:"Scripting_SaveVi.vi"("error in (no error)"=w502, "VIRefToSaveIn"=w503) -> ("error out"=w501:errorcluster)  [unwired: 8 in, 1 out]
            }
            n198 = Unbundle By Name(w493) -> ("Type"=w492:T2)
            n199 = case shown="\"ByViServer\"" w492 {
              tunnel: ["AddClassRefInObjectAttribute" "CloseDown"] -> w498
              frame "ByAggregation", Default {
              }
              frame "ByViServer" {
              }
            }
          }
          frame "AddClassRefInObjectAttribute" {
            w512 = TRUE ("ForceResaving(False)")
            w520 = FALSE ("DeleteAllCurrentAttributesFirst(True)")
            n200 = Unbundle By Name(w519) -> ("BaseInterfaceClassRef"=w530:refnum<vi>, "NewInterfaceClassRef"=w513:refnum<vi>, "ClassName"=w516:string, "SubInterfaceClassName"=w509:string)
            n201 = property class="LVClassLibrary"(reference=w538, error in=w537) -> (reference out=w510:refnum<vi>, error out=w536:errorcluster, "Path"=w535:path)
            n202 = Format Into String(format string="%sRef", w516) -> (resulting string=w517:string)  [unwired: 2 in, 1 out]
            n203 = Build Array(w535) -> (w534:path[])
            n204 = Concatenate Strings("I " ("string"), w509) -> (w523:string)
            n205 = Build Array(w517) -> (w533:string[])
            n206 = Build Array(T8."ClassRefNum" ("DataType")) -> (w531:T15)
            n207 = call <resource>:"Scripting_PlaceControlsInClassAttribute.vi"("ClassRefnum"=w513, "OpenVIWhileEditingAdnRetrunReference"=TRUE, "DeleteAllCurrentAttributesFirst(True)"=w520, "ControlNames"=w533, "DataTypes"=w531, "error in"=w536, "TypeRef"=w534) -> ("Member Data"=w506:refnum<vi>, "error out"=w529:errorcluster)  [unwired: 6 in, 1 out]
            n208 = property class="LVClassLibrary"(reference=w530, error in=w529) -> (error out=w528:errorcluster, "Path"=w527:path)  [unwired: 1 out]
            n209 = Format Into String(format string="%sRef", w523) -> (resulting string=w515:string)  [unwired: 2 in, 1 out]
            n210 = Build Array(w527) -> (w526:path[])
            n211 = Build Array(w515) -> (w522:string[])
            n212 = call <resource>:"Scripting_PlaceControlsInClassAttribute.vi"("ClassRefnum"=w510, "DeleteAllCurrentAttributesFirst(True)"=w520, "ControlNames"=w522, "DataTypes"=w531, "error in"=w528, "TypeRef"=w526) -> ("error out"=w514:errorcluster)  [unwired: 7 in, 2 out]
            n213 = call <resource>:"GDSLvClass_SaveEverythingInClass.vi"("ClassRefIn"=w513, "ForceResaving(False)"=w512, "error in"=w514) -> ("error out"=w511:errorcluster)  [unwired: 15 in, 1 out]
            n214 = call <resource>:"GDSLvClass_SaveEverythingInClass.vi"("ClassRefIn"=w510, "ForceResaving(False)"=w512, "error in"=w511) -> ("error out"=w507:errorcluster)  [unwired: 15 in, 1 out]
            n215 = Bundle By Name(cluster=w519, "RefNameInSubInterface"=w517, "RefNameInClass"=w515) -> (w518:T3)
            n216 = Close Reference(reference=w506, error in (no error)=w507) -> ()  [unwired: 1 out]
          }
          frame "PlaceClassMethodInInterfaceMethod" {
            n217 = Unbundle By Name(w542) -> ("I_MethodRefs"=w547:refnum<vi>[], "C_MethodRefs"=w546:refnum<vi>[])
            n218 = for {
              tunnel: w547 -> [w584] mode=indexing
              tunnel: w546 -> [w583] mode=indexing
              shift-right: [w574] -> w544
              shift-left: w545 -> [w579]
              tunnel: [w548] -> w540 mode=indexing
              w581 = refnum<vi> refnum  # SubVI
              n219 = property class="VI"(reference=w583, error in=w579) -> (error out=w580:errorcluster, "Path"=w582:path)  [unwired: 1 out]
              n220 = property class="VI"(reference=w584, error in=w580) -> (reference out=w575:refnum<vi>, error out=w573:errorcluster, "Diagram"=w577:refnum<vi>, "ConPane"=w570:refnum<vi>)
              n221 = property class="ConPane"(reference=w570) -> (reference out=w557:refnum<vi>, "Ctrls[]"=w560:refnum<vi>[], "TermBnds[]"=w569:T16[])  [unwired: 1 in, 1 out]
              n222 = call <resource>:"Scripting_IndicateConnectorPaneCorners.vi"("TermBnds[]"=w569) -> ("LeftTop"=w568:i32)  [unwired: 7 in, 3 out]
              n223 = Index Array(array=w560, index=w568) -> (element=w556:refnum<vi>)
              n224 = property class="Ctl"(reference=w556) -> ("Terminal"=w555:refnum<vi>)  [unwired: 1 in, 2 out]
              n225 = property class="CtrlTerm"(reference=w555) -> (reference out=w553:refnum<vi>, error out=w554:errorcluster, "Position"=w567:T17)  [unwired: 1 in]
              n226 = Add(x=T9 {"Horizontal"=200, "Vertical"=200} ("relative position/next to refnum"), y=w567) -> (x+y=w565:T17)
              n227 = New VI Object(vi object class=w581, owner refnum=w577, position/next to=w565, 6:w582, 8:w573) -> (object refnum=w572:refnum<vi>, 0:w571:errorcluster)  [unwired: 3 in]
              n228 = property class="SubVI"(reference=w572, error in=w571, "Position"=w565) -> (error out=w562:errorcluster, "Terms[]"=w551:refnum<vi>[])  [unwired: 1 out]
              n229 = call <resource>:"Scripting_IndicateConnectorPaneCorners.vi"("Terminals[]"=w551) -> ("RightTop"=w564:i32, "LeftTop"=w549:i32)  [unwired: 7 in, 2 out]
              n230 = Build Array(w549, w564) -> (w563:i32[])
              n231 = Close Reference(reference=w553, error in (no error)=w554) -> (error out=w552:errorcluster)
              n232 = for {
                tunnel: w551 -> [w587] mode=indexing
                tunnel: w563 -> [w595]
                tunnel: w560 -> [w586] mode=indexing
                shift-right: [w593] -> w561
                shift-left: w562 -> [w592]
                tunnel: w552 -> [_]
                i -> [w594]
                n233 = Search 1D Array(1D array=w595, element=w594) -> (index of element=w591:i32)  [unwired: 1 in]
                n234 = Not A Number/Path/Refnum?(number/path/refnum=w586) -> (NaN/Path/Refnum?=w585:bool)
                n235 = Not A Number/Path/Refnum?(number/path/refnum=w587) -> (NaN/Path/Refnum?=w588:bool)
                n236 = Greater Or Equal To 0?(x=w591) -> (x >= 0?=w589:bool)
                n237 = Compound Arithmetic op=OR(w588, w589, w585) -> (w590:bool)
                n238 = case shown="False" w590 {
                  tunnel: w587 -> [_ w603]
                  tunnel: w586 -> [_ w602]
                  tunnel: [w596 w599] -> w593
                  tunnel: w592 -> [w596 w598]
                  frame True {
                  }
                  frame False {
                    n239 = property class="Ctl"(reference=w602, error in=w598) -> (error out=w597:errorcluster, "Terminal"=w600:refnum<vi>)  [unwired: 1 out]
                    n240 = invoke class="Term" method="Connect Wire"(reference=w603, error in=w597, "Wire Source"=w600, "Auto Wire? (T)"=FALSE) -> (error out=w601:errorcluster)  [unwired: 3 in, 6 out]
                    n241 = Close Reference(reference=w600, error in (no error)=w601) -> (error out=w599:errorcluster)
                  }
                }
              }
              n242 = Close Reference(reference=w572, error in (no error)=w561) -> (error out=w578:errorcluster)
              n243 = Close Reference(reference=w577, error in (no error)=w578) -> (error out=w576:errorcluster)
              n244 = Close Reference(reference=w560, error in (no error)=w561) -> (error out=w559:errorcluster)
              n245 = Delete From Array(array=w551, index=w549) -> (deleted portion=w548:refnum<vi>, array with subset deleted=w550:refnum<vi>[])  [unwired: 1 in]
              n246 = invoke class="VI" method="Save.Instrument"(reference=w575, error in=w576) -> (error out=w574:errorcluster)  [unwired: 4 in, 5 out]
              n247 = Close Reference(reference=w550, error in (no error)=w559) -> (error out=w558:errorcluster)
              n248 = Close Reference(reference=w557, error in (no error)=w558) -> ()  [unwired: 1 out]
            }
            n249 = Bundle By Name(cluster=w542, "SubViUpperLeftTerminal"=w540) -> (w541:T3)
          }
          frame "AddUnBundleInMethods" {
            n250 = Unbundle By Name(w612) -> ("SubViUpperLeftTerminal"=w609:refnum<vi>[], "RefNameInSubInterface"=w608:string, "I_MethodRefs"=w614:refnum<vi>[])
            n251 = Build Array(w608) -> (w607:string[])
            n252 = Bundle(w607) -> (w606:cluster{string[]})  [unwired: 1 in]
            n253 = Build Array(w606) -> (w605:cluster{string[]}[])
            n254 = for {
              tunnel: w614 -> [w616] mode=indexing
              shift-right: [w617] -> w611
              shift-left: w613 -> [w643]
              tunnel: w609 -> [w622] mode=indexing
              tunnel: w605 -> [w632]
              w621 = 2058 items=[".NET Container"=2125, ".NET Refnum"=3441, "2D Picture"=3508, "3D Picture"=23776, "Absolute Value"=1054, "Access Rights"=1412, "ActiveX Container"=2072, "Add"=3915, "Add 1"=1050, "Add Array Elements"=1903, "Agitator"=3831, "AllSpoll"=1960, "Always Copy"=2400, "And"=1061, "And Array Elements"=1911, "Append True/False String"=1511, "Application Refnum"=3412, "Array"=21608, "Array 1"=3300, "Array Constant"=2070, "Array Interface Control"=23777, "Array Max & Min"=1907, "Array Size"=1809, "Array Subset"=2044, "Array To Cluster"=1168, "Array To Spreadsheet String"=1540, "Array of Strings to Path"=1422, "Atmospheric Tank"=3070, "Atmospheric Tank 1"=21751, "Automation Close"=8001, "Automation Open"=8000, "Automation Refnum"=3410, "Avogadro Constant (1/mol)"=23520, "Base 10 Logarithm Of e"=23512, "Bin"=3073, "Bin 1"=21755, "Bitpack to Array"=3135, "Blocking Variable Read"=23786, "Blocking Variable Write"=23789, "Bluetooth Close Connection"=9148, "Bluetooth Create Listener"=9151, "Bluetooth Discover"=9152, "Bluetooth Network Connection Refnum"=3468, "Bluetooth Open Connection"=9153, "Bluetooth Read"=9149, "Bluetooth Wait On Listener"=9147, "Bluetooth Write"=9150, "Boolean Array To Number"=1815, "Boolean To (0,1)"=1167, "Build Array"=2041, "Build Cluster Array"=2047, "Build Matrix"=8500, "Build Path"=1419, "Build Waveform"=2066, "Bundle"=2049, "Bundle By Name"=2057, "Byte Array To String"=1609, "Byte Stream File Refnum"=3408, "CAN Channel"=21966, "CAN Channel 1"=3340, "CAN Channel 2"=2124, "CAN Channel 3"=21817, "CAN Interface"=3339, "CAN Interface 1"=21815, "CAN Interface 2"=2123, "CAN Interface 3"=21964, "CAN Task"=3470, "CAN Task 1"=3471, "CAN Task 2"=21963, "CAN Task 3"=21789, "CPU Information"=24130, "Call By Reference Node"=3901, "Call Chain"=1999, "Call Library Function Node"=2062, "Call Parent Method"=2354, "Cancel Button"=21739, "Cancel Notification"=9107, "Carriage Return Constant"=23500, "Case Structure"=2001, "Cast Unit Bases"=1079, "Check Valve"=3833, "Checkbox"=3117, "Class Specifier Constant"=2094, "Classic Radio Buttons"=22003, "Clear Fixed-Point Overflow Status"=5562, "Close File"=1405, "Close File 1"=8052, "Close Reference"=8011, "Close Variable Connection"=23783, "Cluster"=3400, "Cluster 1"=21607, "Cluster Constant"=2071, "Cluster To Array"=1169, "Code Interface Node"=2050, "Coerce To Type"=2402, "Color Box"=3013, "Color Box Constant"=2120, "Color Box Thin Border"=2905, "Color Ramp"=3022, "Combo Box"=21604, "Combo Box 1"=3304, "Combo Box Constant"=2088, "Complex Conjugate"=1048, "Complex To Polar"=1045, "Complex To Re/Im"=1044, "Compound Arithmetic"=2200, "Compressor"=3832, "Concatenate Strings"=2040, "Conditional Disable Structure"=2064, "Constructor Node"=3904, "Control & Simulation Loop"=2099, "Control Help Window"=1353, "Control Online Help"=1355, "Control Refnum"=3419, "Convert Unit"=2059, "Conveyer"=3827, "Copy"=1416, "Copy 1"=8053, "Cosecant"=1204, "Cosine"=1201, "Cotangent"=1205, "Create Folder"=8055, "Create User Event"=2073, "Current Processor ID"=24131, "Current VI's Menubar"=9000, "Current VI's Path"=1426, "DAQmx Analog Trigger Source"=3336, "DAQmx Analog Trigger Source 1"=2119, "DAQmx Analog Trigger Source 2"=21951, "DAQmx Analog Trigger Source 3"=21774, "DAQmx Device Name"=21773, "DAQmx Device Name 1"=21950, "DAQmx Device Name 2"=2093, "DAQmx Device Name 3"=3318, "DAQmx Global Channel"=3443, "DAQmx Global Channel 1"=21770, "DAQmx Global Channel 2"=21957, "DAQmx Global Channel 3"=3430, "DAQmx Physical Channel"=3335, "DAQmx Physical Channel 1"=21954, "DAQmx Physical Channel 2"=2118, "DAQmx Physical Channel 3"=21777, "DAQmx Scale Name"=21952, "DAQmx Scale Name 1"=21775, "DAQmx Scale Name 2"=3317, "DAQmx Scale Name 3"=2116, "DAQmx Switch"=21953, "DAQmx Switch 1"=3337, "DAQmx Switch 2"=2121, "DAQmx Switch 3"=21776, "DAQmx Task Name"=3442, "DAQmx Task Name 1"=3434, "DAQmx Task Name 2"=21959, "DAQmx Task Name 3"=21778, "DAQmx Terminal"=21955, "DAQmx Terminal 1"=2117, "DAQmx Terminal 2"=21781, "DAQmx Terminal 3"=3319, "Data Cache Size"=24132, "Data Log File Refnum"=3402, "DataSocket Close"=1085, "DataSocket Open"=1084, "DataSocket Read"=1086, "DataSocket Refnum"=3417, "DataSocket Write"=1087, "Date/Time To Seconds"=1308, "Decimal Digit?"=1119, "Decimal String To Number"=1184, "Decimate 1D Array"=2046, "DecomposeArray"=2412, "DecomposeLockDataValRef"=2406, "DecomposeVariant"=2404, "Decrement"=1058, "Default Directory"=1427, "Delete"=8056, "Delete 1"=1417, "Delete Data Value Reference"=2409, "Delete From Array"=3912, "Delete Menu Items"=9004, "Delete Variant Attribute"=8206, "Delete Waveform Attribute"=8209, "Deny Access"=8057, "Dequeue Element"=9113, "Destroy User Event"=2075, "DevClear"=1961, "DevClearList"=1962, "Device Control/Status"=1433, "Device Refnum"=3405, "Diagram Disable Structure"=2054, "Dial"=3050, "Dial 1"=21732, "Digital Data"=3210, "Digital Data 1"=21216, "Digital Waveform Graph"=21718, "Digital Waveform Graph 1"=3511, "Direct Variable Read"=23785, "Direct Variable Write"=23788, "Divide"=1053, "Divide 1"=3918, "Dlg CheckBox"=21924, "Dlg Horiz Scrollbar"=21905, "Dlg Numeric"=2100, "Dlg Numeric 2"=3006, "Dlg String"=2110, "Dlg Vert Scrollbar"=21906, "Down Arrow"=3824, "Down Bow Valve"=3707, "Down Bow Valve 1"=21767, "Down Bow Valve 2"=3807, "Down Rect Valve"=21766, "Down Rect Valve 1"=3706, "Down Rect Valve 2"=3806, "Down Tee"=3818, "Down Tee 1"=3718, "EOF"=1410, "Elementary Charge (C)"=23517, "Empty Array?"=23063, "Empty Path Constant"=23523, "Empty String Constant"=23503, "Empty String/Path?"=1112, "Enable Menu Tracking"=9002, "EnableLocal"=1963, "EnableRemote"=1964, "End of Line Constant"=23525, "Enqueue Element"=9111, "Enqueue Element At Opposite End"=9129, "Enum"=3023, "Enum 1"=21605, "Enum Constant"=2090, "Equal To 0?"=1113, "Equal?"=1102, "Error Ring Constant"=2039, "Event Callback Refnum"=3435, "Event Data Node"=2102, "Event Structure"=2052, "Exchanger"=3828, "Exclusive Or"=1063, "Exponential"=1211, "Exponential (Arg) -1"=1222, "Expression Node"=2201, "FIFO Refnum"=3474, "False Constant"=2006, "Feedback Node, Feedback Node 1"=2353, "FieldPoint IO Point"=21784, "FieldPoint IO Point 1"=3440, "FieldPoint IO Point 2"=3439, "File Dialog"=8058, "File Dialog 1"=8081, "File Path Control"=21730, "File Path Control 1"=3203, "File Path Indicator"=21731, "File Path Indicator 1"=3204, "File/Directory Info"=1413, "File/Directory Info 1"=8082, "FindLstn"=1965, "FindRQS"=1966, "First Call?"=1083, "Fixed-Point Overflow?"=5565, "Fixed-Point to Integer Cast"=5566, "Flat Box"=3602, "Flat Circle"=3605, "Flat Down Triangle"=3623, "Flat Frame"=3608, "Flat Left Triangle"=3620, "Flat Right Triangle"=3621, "Flat Round Button"=3102, "Flat Rounded Box"=3611, "Flat Sequence Structure"=2069, "Flat Square Button"=3103, "Flat Up Triangle"=3622, "Flatten To String"=1164, "Flatten To XML"=8400, "Flattened String To Variant"=8202, "Floating Point Equal?"=23064, "Flush File"=8059, "Flush File 1"=1406, "Flush Queue"=9114, "For Loop"=2002, "Fork"=2194, "Format Date/Time String"=8100, "Format Into File"=2083, "Format Into String"=2081, "Format Value"=1512, "Formula Node"=2004, "Fract/Exp String To Number"=1187, "Framed Color Box"=21019, "Framed Color Box 1"=3008, "Free Label"=2321, "Furnace"=3829, "GPIB Clear"=1954, "GPIB Initialization"=1957, "GPIB Misc"=1956, "GPIB Read"=1951, "GPIB Serial Poll"=1955, "GPIB Status"=1959, "GPIB Trigger"=1953, "GPIB Wait"=1958, "GPIB Write"=1950, "Gauge"=21009, "Gauge 1"=3040, "Generate Front Panel Activity"=1329, "Generate Occurrence"=1700, "Generate User Event"=2074, "Generate User-Defined Trace Event"=2250, "Get Datalog Position"=8061, "Get Date/Time In Seconds"=1303, "Get Date/Time String"=1600, "Get Drag Drop Data"=9154, "Get File Position"=8062, "Get File Size"=8063, "Get Fixed-Point Components"=11163, "Get Help Window Status"=1354, "Get Matrix Diagonal"=8501, "Get Matrix Elements"=8502, "Get Menu Item Info"=9005, "Get Menu Selection"=9001, "Get Menu Short Cut Info"=9007, "Get Notifier Status"=9103, "Get Number of Records"=8064, "Get Permissions"=8065, "Get Queue Status"=9110, "Get Submatrix"=8503, "Get Type and Creator"=8066, "Get Variant Attribute"=8205, "Get Volume Info"=8067, "Get Waveform Attribute"=8208, "Get Waveform Components"=2067, "Global Variable"=2060, "Gravitational Constant (N m2/kg2)"=23519, "Greater Or Equal To 0?"=1114, "Greater Or Equal?"=1103, "Greater Than 0?"=1117, "Greater?"=1110, "Handle Peek"=1604, "Handle Poke"=1605, "Hex Digit?"=1123, "Hexadecimal String To Number"=1185, "Hopper"=21754, "Hopper 1"=3072, "Horiz Line"=3821, "Horiz Pipe"=3710, "Horiz Pipe 1"=3810, "Horizontal Button Box"=3636, "Horizontal Fill Slide"=3012, "Horizontal Fill Slide 1"=21100, "Horizontal Graduated Bar"=21106, "Horizontal Pointer Slide"=21101, "Horizontal Pointer Slide 1"=3011, "Horizontal Progress Bar"=21102, "Horizontal Scrollbar"=21110, "Horizontal Slide"=3010, "Horizontal Slide Switch"=3114, "Horizontal Smooth Box"=3633, "Horizontal Splitter Bar"=21861, "Horizontal Splitter Bar (Classic)"=21863, "Horizontal Splitter Bar (System)"=21865, "Horizontal Switch"=3108, "Horizontal Tank"=3071, "Horizontal Toggle Switch"=3110, "Horizontal Toggle Switch 1"=21700, "Hyperbolic Cosecant"=23053, "Hyperbolic Cosine"=1215, "Hyperbolic Cotangent"=23055, "Hyperbolic Secant"=23054, "Hyperbolic Sine"=1214, "Hyperbolic Tangent"=1216, "IMAQ Session"=3415, "IP To String"=1710, "IVI Delete Session"=8103, "IVI Logical Name"=3420, "IVI Logical Name 1"=3414, "IVI Logical Name 2"=21736, "IVI New Session"=8102, "Implies"=1080, "In Place Element Structure"=2360, "In Range and Coerce"=1127, "Include Fixed-Point Overflow Status"=5564, "Increment"=1057, "Index & Bundle Cluster Array"=2056, "Index Array"=2042, "Index String Array"=1531, "Initialize Array"=2053, "Inline C Node"=2104, "Insert Into Array"=3911, "Insert Menu Items"=9003, "Integer to Fixed-Point Cast"=5567, "Intensity Chart"=21719, "Intensity Chart 1"=3509, "Intensity Graph"=21720, "Intensity Graph 1"=3510, "Interleave 1D Arrays"=2045, "Interpolate 1D Array"=1905, "Inverse Cosecant"=23050, "Inverse Cosine"=1207, "Inverse Cotangent"=23052, "Inverse Hyperbolic Cosecant"=23056, "Inverse Hyperbolic Cosine"=1218, "Inverse Hyperbolic Cotangent"=23058, "Inverse Hyperbolic Secant"=23057, "Inverse Hyperbolic Sine"=1217, "Inverse Hyperbolic Tangent"=1219, "Inverse Secant"=23051, "Inverse Sine"=1206, "Inverse Tangent"=1208, "Inverse Tangent (2 Input)"=1228, "Invoke Node"=3900, "IrDA Close Connection"=9144, "IrDA Create Listener"=9140, "IrDA Discover"=9141, "IrDA Network Connection Refnum"=3450, "IrDA Open Connection"=9142, "IrDA Read"=9145, "IrDA Wait On Listener"=9143, "IrDA Write"=9146, "Join"=2195, "Join Numbers"=1171, "Junction"=2197, "Knob"=21000, "Knob 1"=3005, "LED Button"=3116, "LabVIEW Object"=3457, "Label"=21960, "Labeled Oblong Button"=3125, "Labeled Rectangular Button"=3124, "Labeled Round Button"=3122, "Labeled Square Button"=3123, "Leak Variant Value Reference"=2410, "Left Arrow"=3826, "Left Bow Valve"=3701, "Left Bow Valve 1"=3801, "Left Bow Valve 2"=21761, "Left Down Elbow"=3711, "Left Down Elbow 1"=3811, "Left Pump"=3713, "Left Pump 1"=3813, "Left Rect Valve"=3700, "Left Rect Valve 1"=21760, "Left Rect Valve 2"=3800, "Left Tee"=3709, "Left Tee 1"=3809, "Left Up Elbow"=3808, "Left Up Elbow 1"=3708, "Less Or Equal To 0?"=1115, "Less Or Equal?"=1104, "Less Than 0?"=1118, "Less?"=1111, "Lexical Class"=1126, "Line Feed Constant"=23501, "List Directory"=1418, "List Folder"=8083, "Listbox"=21792, "Listbox 1"=21806, "Listbox Symbol Ring Constant"=2038, "Local Variable"=2061, "Lock Range"=1411, "Logarithm Base 10"=1210, "Logarithm Base 2"=1225, "Logarithm Base X"=1224, "Logical Shift"=1081, "Lossy Enqueue Element"=9130, "Lowered Rounded Box"=3638, "MATLAB script"=9020, "Machine Epsilon"=23528, "MakeAddr"=1967, "Mantissa & Exponent"=1150, "Match First String"=1532, "Match Pattern"=1535, "Match True/False String"=1533, "MathScript Call By Reference Node"=3906, "MathScript Node"=2357, "Matrix Size"=8507, "Max & Min"=1108, "Menu Refnum"=3413, "Menu Ring"=3018, "Menu Ring 1"=21600, "Menu-Popup Ring"=3017, "Merge Signals"=2350, "Meter"=21008, "Meter 1"=3030, "Mixed Signal Graph"=21721, "Molar Gas Constant (J/(mol K))"=23522, "Motion Resource"=21787, "Motion Resource 1"=3448, "Motion Resource 2"=3449, "Motor"=3720, "Motor 1"=3820, "Move"=1415, "Move 1"=8068, "Multi-Segment Pipe"=23780, "Multicolumn Listbox"=21799, "Multicolumn Listbox 1"=21791, "Multiple Selection Listbox"=3208, "Multiply"=1052, "Multiply 1"=3917, "Multiply Array Elements"=1904, "Multirate Structure"=2199, "Natural Logarithm"=1209, "Natural Logarithm (Arg +1)"=1221, "Natural Logarithm Base"=23510, "Natural Logarithm Of 10"=23513, "Natural Logarithm Of 2"=23514, "Natural Logarithm Of Pi"=23508, "Negate"=1069, "Negative Infinity"=23509, "New Data Value Reference"=2408, "New Directory"=1402, "New File"=1404, "New VI"=8014, "New VI Object"=8015, "Not"=1064, "Not A Number/Path/Refnum?"=1128, "Not A Path Constant"=23524, "Not And"=1071, "Not Equal To 0?"=1116, "Not Equal?"=1105, "Not Exclusive Or"=1073, "Not Or"=1072, "Not a Refnum Constant"=23526, "Not a Shared Variable"=23527, "Notifier Refnum"=3423, "Number To Boolean Array"=1814, "Number To Decimal String"=1180, "Number To Engineering String"=1183, "Number To Exponential String"=1505, "Number To Fractional String"=1506, "Number To Hexadecimal String"=1181, "Number To Octal String"=1182, "Number of Cache Levels"=24133, "Numeric Constant"=2005, "Numeric Control"=3000, "Numeric Control 1"=21003, "Numeric Indicator"=3001, "Numeric Indicator 1"=21004, "OK Button"=21738, "OLE Variant"=3150, "Obtain Notifier"=9101, "Obtain Queue"=9108, "Occurrence Refnum"=3406, "Octal Digit?"=1129, "Octal String To Number"=1186, "Old VISA Open"=1921, "One Button Dialog"=1340, "Open Application Reference"=8012, "Open Device"=1430, "Open File"=1403, "Open Tank"=21752, "Open Tank 1"=3074, "Open VI Object Reference"=8013, "Open VI Reference"=8010, "Open Variable Connection"=23779, "Open Variable Connection in Background"=23791, "Open and Verify Variable Connection"=23790, "Open/Create/Replace Datalog"=8054, "Open/Create/Replace File"=8050, "Or"=1062, "Or Array Elements"=1910, "PPoll"=1969, "PPollConfig"=1970, "PPollUnconfig"=1971, "Package Matrix"=23001, "PassControl"=1968, "Path Constant"=2009, "Path To String"=1077, "Path Type"=1421, "Path to Array of Strings"=1423, "Pi"=23504, "Pi Divided By 2"=23506, "Pi Multiplied By 2"=23505, "Pick Line"=1510, "Pict Ring"=21602, "Pict Ring 1"=3015, "PixMap"=3505, "PixMap (Do not touch it!!)"=3507, "Planck's Constant (J/Hz)"=23516, "Platform Flat Square Button"=3134, "Plug-In Control"=21820, "Polar To Complex"=1047, "Polar To Re/Im"=23061, "Positive Infinity"=23515, "Power Of 10"=1212, "Power Of 2"=1223, "Power Of X"=1213, "Preserve Run-Time Class"=8018, "Pressure Tank"=3075, "Pressure Tank 1"=21753, "Preview Queue Element"=9112, "Printable?"=1124, "Property Node"=1920, "Pulldown Menu Ring"=3061, "Push Button"=21001, "Queue Refnum"=3424, "Quit LabVIEW"=1352, "Quotient & Remainder"=1056, "RT FIFO Create"=24000, "RT FIFO Delete"=24003, "RT FIFO Read"=24001, "RT FIFO Write"=24002, "Radio Buttons"=22001, "Raised Box"=3600, "Raised Box 1"=3637, "Raised Circle"=3603, "Raised Down Triangle"=3615, "Raised Frame"=3606, "Raised Left Triangle"=3612, "Raised Right Triangle"=3613, "Raised Rounded Box"=3609, "Raised Up Triangle"=3614, "Random Number (0-1)"=1070, "RcvRespMsg"=1972, "Re/Im To Complex"=1046, "Re/Im To Polar"=23060, "Read Datalog"=8069, "Read Device"=1432, "Read File"=1407, "Read Variable"=23781, "Read from Binary File"=8051, "Read from Text File"=8070, "ReadStatus"=1973, "Receive"=1974, "ReceiveSetup"=1975, "Recessed Box"=3601, "Recessed Circle"=3604, "Recessed Down Triangle"=3619, "Recessed Frame"=3607, "Recessed Left Triangle"=3616, "Recessed Menu Ring"=3019, "Recessed Right Triangle"=3617, "Recessed Rounded Box"=3610, "Recessed Up Triangle"=3618, "Reciprocal"=1059, "Reciprocal Of Pi"=23507, "Reciprocal Of e"=23511, "RecomposeArray"=2403, "RecomposeUnlockDataValRef"=2407, "RecomposeVariant"=2405, "Rectangular Stop Button"=3128, "Refnum to Path"=1424, "Refnum to Session"=2306, "Region"=2196, "Register Event Callback"=2078, "Register For Events"=2065, "Register Session"=2319, "Release Notifier"=9102, "Release Queue"=9109, "Remove Fixed-Point Overflow Status"=5563, "Replace Array Subset"=3910, "Replace Substring"=3913, "Request Deallocation"=1610, "ResetSys"=1976, "Reshape Array"=2055, "Resize Matrix"=8508, "Reverse 1D Array"=1900, "Reverse String"=1537, "Right Arrow"=3825, "Right Bow Valve"=21765, "Right Bow Valve 1"=3705, "Right Bow Valve 2"=3805, "Right Down Elbow"=3817, "Right Down Elbow 1"=3717, "Right Pump"=3719, "Right Pump 1"=3819, "Right Rect Valve"=3804, "Right Rect Valve 1"=3704, "Right Rect Valve 2"=21764, "Right Tee"=3715, "Right Tee 1"=3815, "Right Up Elbow"=3814, "Right Up Elbow 1"=3714, "Ring Constant"=2008, "Rocker"=21002, "Rotary Feeder"=3830, "Rotate"=1082, "Rotate 1D Array"=1906, "Rotate Left With Carry"=1606, "Rotate Right With Carry"=1607, "Rotate String"=1536, "Round Button"=3100, "Round LED"=3120, "Round LED 1"=21012, "Round Light"=3104, "Round Push Button"=3112, "Round Push Button 2"=3118, "Round Radio Button"=3106, "Round Stop Button"=3127, "Round To Nearest"=1055, "Round Toward +Infinity"=1076, "Round Toward -Infinity"=1075, "Rydberg Constant (1/m)"=23521, "Scale By Power Of 2"=1074, "Scan From File"=2082, "Scan From String"=2080, "Scan String For Tokens"=8101, "Scan Value"=1534, "Scanned Variable Read"=23784, "Scanned Variable Write"=23787, "Search 1D Array"=1901, "Search and Replace String"=3914, "Search/Split String"=1538, "Secant"=1203, "Seconds To Date/Time"=1309, "Seek"=1409, "Select"=1516, "Send"=1977, "Send Notification"=9104, "SendCmds"=1978, "SendDataBytes"=1979, "SendIFC"=1980, "SendLLO"=1982, "SendList"=1981, "SendSetup"=1983, "Session to Refnum"=2307, "Set Datalog Position"=8072, "Set File Position"=8073, "Set File Size"=8074, "Set Matrix Diagonal"=8504, "Set Matrix Elements"=8505, "Set Menu Item Info"=9006, "Set Number of Records"=8075, "Set Occurrence"=1702, "Set Permissions"=8076, "Set Submatrix"=8506, "Set Type and Creator"=8077, "Set Variant Attribute"=8204, "Set Waveform Attribute"=8207, "SetRWLS"=1984, "SetTimeOut"=1985, "Shared Variable"=23778, "Shared Variable Constant"=3473, "Shared Variable Control"=3472, "Shared Variable Control 1"=21814, "Shared Variable to String"=1831, "Sign"=1049, "Simple Horizontal Slide"=3003, "Simple Numeric"=3029, "Simple Numeric 1"=2900, "Simple String"=2115, "Simple Vertical Slide"=3002, "Sinc"=1227, "Sine"=1200, "Sine & Cosine"=1220, "Size Handle"=1603, "Slide Switch"=21011, "Sort 1D Array"=1120, "Sort Array of String, Sort Array of String 1"=23065, "Speed Of Light In Vacuum (m/sec)"=23518, "Split 1D Array"=1908, "Split Button"=21020, "Split Number"=1170, "Split Signals"=2351, "Spreadsheet String To Array"=1539, "Square"=23059, "Square Button"=3101, "Square LED"=3121, "Square LED 1"=21013, "Square Light"=3105, "Square Push Button"=3113, "Square Push Button 2"=3119, "Square Radio Button"=3107, "Square Root"=1060, "Stacked Sequence Structure"=2000, "State"=2198, "State Diagram"=2051, "Static VI Reference"=2084, "Stop"=1350, "Stop Button"=21230, "String Constant"=2007, "String Control"=3200, "String Control 1"=21701, "String Indicator"=3201, "String Indicator 1"=21702, "String Length"=1502, "String Subset"=1503, "String To Byte Array"=1608, "String To IP"=1711, "String To Path"=1078, "String to Shared Variable"=1830, "Strip Path"=1420, "SubPanel"=21810, "SubPanel (Classic)"=21811, "SubPanel (System)"=21823, "Subtract"=1051, "Subtract 1"=3916, "Swap Bytes"=1162, "Swap Values"=2401, "Swap Vector Element"=1912, "Swap Words"=1163, "System Button"=3130, "System Cancel Button"=3131, "System Checkbox"=3132, "System Chiseled Line"=3632, "System Colored Rectangle"=3625, "System Combo Box"=21917, "System Enum"=3062, "System Horizontal Pointer Slide"=21902, "System Horizontal Progress Bar"=21910, "System Horizontal Slide"=21904, "System Label"=21961, "System Listbox"=21805, "System Mixed Checkbox"=21333, "System Multicolumn Listbox"=21798, "System Numeric"=21919, "System Path Control"=21922, "System Pict Ring"=21925, "System Radio Button"=3133, "System Radio Buttons"=22002, "System Recessed Frame"=3624, "System Ring"=3060, "System Spin Control"=21900, "System String"=21920, "System Tab Control"=3331, "System Table"=21797, "System Time Stamp"=21967, "System Tree"=21794, "System Vertical Pointer Slide"=21901, "System Vertical Progress Bar"=21909, "System Vertical Slide"=21903, "TCP Close Connection"=1713, "TCP Create Listener"=1717, "TCP Flattened Read"=1718, "TCP Flattened Write"=1719, "TCP Flex Read"=1720, "TCP Flex Write"=1721, "TCP Network Connection Refnum"=3407, "TCP Open Connection"=1715, "TCP Read"=1716, "TCP Wait On Listener"=1712, "TCP Write"=1714, "TDMS Close"=24113, "TDMS Defragment"=24119, "TDMS File"=3477, "TDMS Flush"=24117, "TDMS Get Properties"=24115, "TDMS List Contents"=24116, "TDMS Open"=24112, "TDMS Read"=24111, "TDMS Refnum To File ID"=24120, "TDMS Set Properties"=24114, "TDMS Write"=24110, "TDMS Write IP"=24118, "Tab Constant"=23502, "Tab Control"=3330, "Tab Control 1"=3332, "Table"=21796, "Table 1"=21790, "Tag Attribute Ring"=2063, "Tangent"=1202, "Tank"=21006, "Tank 1"=3020, "Temporary Directory"=1435, "TestSRQ"=1986, "TestSys"=1987, "Text & Pict Ring"=21603, "Text & Pict Ring 1"=3016, "Text Button"=21015, "Text Ring"=21601, "Text Ring 1"=3014, "Text to UTF-8"=23066, "Thermometer"=21007, "Thermometer 1"=3021, "Thick Chiseled Line"=3630, "Thick Line"=3629, "Thick Line with Arrow"=3631, "Thick Lowered Box"=3635, "Thin Chiseled Line"=3627, "Thin Line"=3626, "Thin Line with Arrow"=3628, "Threshold 1D Array"=1909, "Tick Count (ms)"=1300, "Time Stamp Constant"=2068, "Time Stamp Control"=21913, "Time Stamp Control 1"=5555, "Time Stamp Indicator"=21914, "Time Stamp Indicator 1"=5556, "Timed Loop"=5570, "Timed Sequence"=5573, "To Byte Integer"=1140, "To Double Precision Complex"=1152, "To Double Precision Float"=1147, "To Extended Precision Complex"=1154, "To Extended Precision Float"=1149, "To Fixed-Point"=5561, "To Long Integer"=1142, "To Lower Case"=1189, "To More Generic Class"=8017, "To More Specific Class"=8016, "To OLE Variant"=8002, "To Probe String"=2413, "To Quad Integer"=1155, "To Single Precision Complex"=1151, "To Single Precision Float"=1146, "To Time Stamp"=5560, "To Unsigned Byte Integer"=1143, "To Unsigned Long Integer"=1145, "To Unsigned Quad Integer"=1156, "To Unsigned Word Integer"=1144, "To Upper Case"=1188, "To Variant"=8201, "To Word Integer"=1141, "Traditional DAQ Channel"=21733, "Traditional DAQ Channel 1"=2085, "Traditional DAQ Channel 2"=3320, "Transpose 1D Array"=23068, "Transpose 2D Array"=1902, "Transpose Matrix"=8509, "Tree"=21819, "Tree 1"=21793, "Trigger"=1988, "TriggerList"=1989, "Two Button Dialog"=1341, "Type Cast"=1166, "Type and Creator"=1434, "UDP Close"=1726, "UDP Multicast Open"=1727, "UDP Network Connection Refnum"=3418, "UDP Open"=1723, "UDP Read"=1724, "UDP Write"=1725, "UTF-8 to Text"=23067, "Unbitpack from Array"=3136, "Unbundle"=2048, "Unbundle By Name"=2058, "Unflatten From String"=1165, "Unflatten From XML"=8401, "Unleak Variant Value Reference"=2411, "Unpackage Matrix"=23000, "Unregister For Events"=2076, "Unregister Session"=2320, "Up Arrow"=3823, "Up Bow Valve"=3703, "Up Bow Valve 1"=3803, "Up Bow Valve 2"=21763, "Up Rect Valve"=3702, "Up Rect Valve 1"=21762, "Up Rect Valve 2"=3802, "Up Tee"=3712, "Up Tee 1"=3812, "User Defined Refnum"=3428, "User Defined Refnum Tag"=21745, "User Defined Refnum Tag 1"=3429, "User Defined Refnum Tag Constant"=3426, "User Defined Refnum Tag Flatten"=21747, "User Defined Refnum Tag Flatten 1"=3454, "User Defined Tag"=21749, "User Defined Tag 1"=3329, "User Defined Tag Constant"=2114, "User Item"=3506, "VI Library"=1425, "VI Refnum"=3422, "VI Server Reference"=2091, "VISA Assert Interrupt Signal"=2309, "VISA Assert Trigger"=1929, "VISA Assert Utility Signal"=2310, "VISA Clear"=1927, "VISA Close"=1922, "VISA Disable Event"=1940, "VISA Discard Events"=1941, "VISA Enable Event"=1942, "VISA Find Resource"=1923, "VISA Flush I/O Buffer"=2302, "VISA GPIB Command"=2315, "VISA GPIB Control ATN"=2316, "VISA GPIB Control REN"=2304, "VISA GPIB Pass Control"=2317, "VISA GPIB Send IFC"=2318, "VISA In 16"=1930, "VISA In 32"=1944, "VISA In 64"=2140, "VISA In 8"=1936, "VISA Lock"=1993, "VISA Map Address"=1932, "VISA Map Trigger"=2311, "VISA Memory Allocation"=1997, "VISA Memory Allocation Ex"=2146, "VISA Memory Free"=1998, "VISA Move"=2303, "VISA Move In 16"=1948, "VISA Move In 32"=1991, "VISA Move In 64"=2144, "VISA Move In 8"=1946, "VISA Move Out 16"=1949, "VISA Move Out 32"=1992, "VISA Move Out 64"=2145, "VISA Move Out 8"=1947, "VISA Open"=2308, "VISA Out 16"=1931, "VISA Out 32"=1945, "VISA Out 64"=2141, "VISA Out 8"=1937, "VISA Peek 16"=1934, "VISA Peek 32"=1995, "VISA Peek 64"=2142, "VISA Peek 8"=1938, "VISA Poke 16"=1935, "VISA Poke 32"=1996, "VISA Poke 64"=2143, "VISA Poke 8"=1939, "VISA Read"=1925, "VISA Read STB"=1928, "VISA Read To File"=2313, "VISA Refnum to Session"=2300, "VISA Resource Name"=3421, "VISA Set I/O Buffer Size"=2301, "VISA Status Description"=1924, "VISA USB Control In"=2086, "VISA USB Control Out"=2087, "VISA Unlock"=1994, "VISA Unmap Address"=1933, "VISA Unmap Trigger"=2312, "VISA VXI Cmd or Query"=2305, "VISA Wait on Event"=1943, "VISA Write"=1926, "VISA Write From File"=2314, "VISA resource name"=3409, "VISA resource name 1"=21737, "Variable Class Specifier Constant"=2106, "Variable Configuration"=3475, "Variant"=3310, "Variant To Data"=8003, "Variant To Flattened String"=8203, "Vert Line"=3822, "Vert Pipe"=3816, "Vert Pipe 1"=3716, "Vert Rocker"=21740, "Vertical Fill Slide"=21014, "Vertical Fill Slide 1"=3009, "Vertical Graduated Bar"=21107, "Vertical Pointer Slide"=21017, "Vertical Pointer Slide 1"=3007, "Vertical Progress Bar"=21104, "Vertical Scrollbar"=21111, "Vertical Slide"=3004, "Vertical Slide Switch"=21741, "Vertical Slide Switch 1"=3115, "Vertical Smooth Box"=3634, "Vertical Splitter Bar"=21860, "Vertical Splitter Bar (Classic)"=21862, "Vertical Splitter Bar (System)"=21864, "Vertical Switch"=3109, "Vertical Toggle Switch"=21005, "Vertical Toggle Switch 1"=3111, "Volume Info"=1414, "Wait (ms)"=1302, "Wait For Activity"=1722, "Wait For Front Panel Activity"=1328, "Wait Until Next ms Multiple"=1327, "Wait for GPIB RQS"=1952, "Wait on Notification"=9105, "Wait on Notification from Multiple"=9106, "Wait on Notification from Multiple with Notifier History"=9132, "Wait on Notification with Notifier History"=9131, "Wait on Occurrence"=1701, "WaitSRQ"=1990, "Waveform Chart"=21010, "Waveform Chart 1"=3501, "Waveform Chart 2"=21717, "Waveform Graph"=21703, "Waveform Graph 1"=3504, "While Loop"=2003, "While Loop 1"=2352, "White Space?"=1125, "Write Datalog"=8079, "Write Device"=1431, "Write File"=1408, "Write Variable"=23782, "Write to Binary File"=8078, "Write to Text File"=8080, "XY Graph"=21716, "XY Graph 1"=3500, "Y-th Root of X"=23062]
              w651 = refnum<vi> refnum  # NamedUnbundler
              n255 = property class="VI"(reference=w616, "BDWin.Open"=FALSE ("Block Diagram Window:Open")) -> ()  [unwired: 1 in, 2 out]
              n256 = property class="VI"(reference=w616, error in=w643) -> (error out=w650:errorcluster, "Diagram"=w620:refnum<vi>, "ConPane"=w649:refnum<vi>)  [unwired: 1 out]
              n257 = property class="ConPane"(reference=w649) -> (reference out=w626:refnum<vi>, "Ctrls[]"=w624:refnum<vi>[], "TermBnds[]"=w648:T16[])  [unwired: 1 in, 1 out]
              n258 = call <resource>:"Scripting_IndicateConnectorPaneCorners.vi"("TermBnds[]"=w648) -> ("LeftTop"=w647:i32)  [unwired: 7 in, 3 out]
              n259 = Index Array(array=w624, index=w647) -> (element=w644:refnum<vi>)
              n260 = property class="Ctl"(reference=w644) -> ("Terminal"=w642:refnum<vi>)  [unwired: 1 in, 2 out]
              n261 = property class="CtrlTerm"(reference=w642) -> (reference out=w623:refnum<vi>, error out=w627:errorcluster, "Position"=w641:T17)  [unwired: 1 in]
              n262 = Add(x=T9 {"Horizontal"=100, "Vertical"=100} ("relative position/next to refnum"), y=w641) -> (x+y=w645:T17)
              n263 = New VI Object(vi object class=w651, owner refnum=w620, style=w621, position/next to=w645, 8:w650) -> (object refnum=w639:refnum<vi>, 0:w638:errorcluster)  [unwired: 3 in]
              n264 = property class="NmdUnbndl"(reference=w639, error in=w638, "FullElemNms[]"=w632) -> (reference out=w629:refnum<vi>, error out=w636:errorcluster, "Terms[]"=w631:refnum<vi>[])
              n265 = Index Array(array=w631) -> (element #1=w637:refnum<vi>, element #2=w633:refnum<vi>)  [unwired: 2 in]
              n266 = Close Reference(reference=w626, error in (no error)=w627) -> (error out=w625:errorcluster)
              n267 = invoke class="Term" method="Connect Wire"(reference=w637, error in=w636, "Wire Source"=w623, "Auto Wire? (T)"=FALSE) -> (error out=w634:errorcluster)  [unwired: 3 in, 6 out]
              n268 = Close Reference(reference=w624, error in (no error)=w625) -> ()  [unwired: 1 out]
              n269 = invoke class="Term" method="Connect Wire"(reference=w633, error in=w634, "Wire Source"=w622, "Auto Wire? (T)"=FALSE) -> (error out=w618:errorcluster)  [unwired: 3 in, 6 out]
              n270 = disable-structure shown="Enabled" {
                disable-tunnel: w620 -> [w655 _]
                disable-tunnel: [w654 w656] -> w619
                disable-tunnel: w618 -> [w653 w656]
                frame Disabled {
                  w652 = T18 {"Alignment"=enum."Center", "Rules"=enum."Strict", "Max Heuristic Iterations"=5, "Max Simplex Iterations"=5, "Block Padding"={"Horizontal"=16, "Vertical"=16}, "Wire Padding"={"Horizontal"=10, "Vertical"=10}, "Auto-Tune by Topology"=FALSE, "Fine-Tune Y Positions"=FALSE, "Align All Controls on Left"=TRUE, "Align All Indicators on Right"=TRUE, "Use Array Dimension Heuristics"=FALSE} ("Clean Up Options")
                  n271 = invoke class="TopLvlDiag" method="CleanUp"(reference=w655, error in=w653) -> (error out=w654:errorcluster)  [unwired: 2 in, 3 out]
                }
                frame Enabled {
                }
              }
              n272 = invoke class="VI" method="Save.Instrument"(reference=w616, error in=w619) -> (error out=w617:errorcluster)  [unwired: 4 in, 5 out]
              n273 = Close Reference(reference=w631, error in (no error)=w617) -> (error out=w630:errorcluster)
              n274 = Close Reference(reference=w623, error in (no error)=w617) -> ()  [unwired: 1 out]
              n275 = Close Reference(reference=w622, error in (no error)=w617) -> ()  [unwired: 1 out]
              n276 = Close Reference(reference=w629, error in (no error)=w630) -> (error out=w628:errorcluster)
              n277 = Close Reference(reference=w620, error in (no error)=w628) -> ()  [unwired: 1 out]
            }
          }
          frame "CreateGetRefMethod" {
            w678 = refnum<vi> refnum  # NamedUnbundler
            n278 = Unbundle By Name(w665) -> ("RefNameInClass"=w669:string, "BaseInterfaceClassRef"=w673:refnum<vi>)
            n279 = Unbundle By Name(w665) -> ("Application"=w698:refnum<vi>, "GetRefVI"=w705:path, "BaseInterfaceName"=w700:string)
            n280 = property class="LVClassLibrary"(reference=w704) -> (reference out=w686:refnum<vi>, "Path"=w703:path)  [unwired: 1 in, 1 out]
            n281 = Strip Path(path=w703) -> (stripped path=w699:path)  [unwired: 1 out]
            n282 = Format Into String(format string="GetI_%s.vi", w700) -> (resulting string=w701:string)  [unwired: 2 in, 1 out]
            n283 = call <resource>:"GDSLvClass_GetClassInfo.vi"("Class Refnum In"=w673, "error in (no error)"=w691) -> ("ClassMemberPath"=w689:path, "error out"=w690:errorcluster)  [unwired: 14 in, 2 out]
            n284 = Build Path(base path=w699, name or relative path=w701) -> (appended path=w661:path)
            n285 = call <resource>:"GDSLvClass_GetClassInfo.vi"("Class Refnum In"=w686, "error in (no error)"=w690) -> ("Class Refnum Out"=w685:refnum<vi>, "ClassMemberPath"=w688:path, "error out"=w692:errorcluster)  [unwired: 14 in, 1 out]
            n286 = Copy(8:w692, 10:w661, 11:w705) -> (0:w663:errorcluster)  [unwired: 2 in, 2 out]
            n287 = Set Permissions(7:i16 511 ("permissions"), 8:w663, 11:w661) -> (0:w662:errorcluster, 3:w660:path)  [unwired: 2 in]
            n288 = Open VI Reference(application reference (local)=w698, vi path=w660, error in (no error)=w662) -> (vi reference=w682:refnum<vi>, error out=w696:errorcluster)  [unwired: 3 in]
            n289 = Build Array(w669) -> (w672:string[])
            n290 = Bundle(w672) -> (w671:cluster{string[]})  [unwired: 1 in]
            n291 = property class="VI"(reference=w682, error in=w696) -> (reference out=w666:refnum<vi>, error out=w683:errorcluster, "Panel"=w697:refnum<vi>)
            n292 = Build Array(w671) -> (w670:cluster{string[]}[])
            n293 = property class="Pnl"(reference=w697, error in=w683) -> (reference out=w684:refnum<vi>, error out=w694:errorcluster, "Controls[]"=w695:refnum<vi>[])
            n294 = Bundle By Name(cluster=w665, "GetVIRef"=w666) -> (w664:T3)
            n295 = for {
              tunnel: w695 -> [w715] mode=indexing
              shift-right: [w710] -> w693
              shift-left: w694 -> [w712]
              tunnel: w689 -> [w708]
              tunnel: w688 -> [w707]
              n296 = property class="Ctl"(reference=w715, error in=w712) -> (reference out=w709:refnum<vi>, error out=w711:errorcluster, "Label.Text"=w714:string, "ClassName"=w713:string)
              n297 = case shown="\"LabVIEWClassControl\"" w713 {
                tunnel: w714 -> [_ w727]
                tunnel: [w717 w721] -> w710
                tunnel: w711 -> [w717 w722]
                tunnel: w709 -> [w716 w724]
                tunnel: w708 -> [_ w719]
                tunnel: w707 -> [_ w718]
                frame "False", Default {
                  n298 = Close Reference(reference=w716) -> ()  [unwired: 1 in, 1 out]
                }
                frame "LabVIEWClassControl" {
                  n299 = Equal?(x=w727, y="InterfaceOut") -> (x = y?=w725:bool)
                  n300 = Select(t=w719, s=w725, f=w718) -> (s? t:f=w720:path)
                  n301 = invoke class="Ctl" method="Replace"(reference=w724, error in=w722, "Path"=w720) -> (reference out=w723:refnum<vi>, error out=w721:errorcluster)  [unwired: 3 in, 4 out]
                  n302 = Close Reference(reference=w723) -> ()  [unwired: 1 in, 1 out]
                }
              }
            }
            n303 = Close Reference(reference=w684, error in (no error)=w693) -> (error out=w667:errorcluster)
            n304 = call <resource>:"Scripting_FindNodeOnDiagram.vi"("ViRef(Ignored If Not Wired)"=w682, "NodeTypesToSearchFor"=string[] ["NamedUnbundler"], "error in (no error)"=w667) -> ("Nodes"=w674:refnum<vi>[], "error out"=w679:errorcluster)  [unwired: 15 in]
            n305 = Index Array(array=w674) -> (element=w680:refnum<vi>)  [unwired: 1 in]
            n306 = To More Specific Class(target class=w678, reference=w680, error in=w679) -> (specific class reference=w677:refnum<vi>, error out=w676:errorcluster)
            n307 = property class="NmdUnbndl"(reference=w677, error in=w676, "FullElemNms[]"=w670) -> (error out=w675:errorcluster)  [unwired: 1 out]
            n308 = Close Reference(reference=w674, error in (no error)=w675) -> (error out=w668:errorcluster)
            n309 = invoke class="LVClassLibrary" method="AddFile"(reference=w685, error in=w668, "Path"=w661) -> (error out=w658:errorcluster)  [unwired: 1 in, 3 out]
            n310 = call <resource>:"CommonVIs_Wait.vi"("error in"=w658) -> ("error out"=w657:errorcluster)  [unwired: 9 in]
            n311 = invoke class="VI" method="Save.Instrument"(reference=w666, error in=w657) -> (error out=w687:errorcluster)  [unwired: 4 in, 5 out]
          }
          frame "UpdateGetRefIcon" {
            n312 = property class="LVClassLibrary" props=["Path", "Member Data"](reference=w752, error in=w751) -> (error out=w749:errorcluster, "Member Data"=w729:refnum<vi>)  [unwired: 2 out]
            n313 = Unbundle By Name(w753) -> ("GetVIRef"=w734:refnum<vi>)
            n314 = call <resource>:"GDSLvIcon_AnalyseViIcon.vi"("ViRef/LvCLassRef/LvLibRef/ViPath"=w729, "error in (no error)"=w749) -> ("FrameColor"=w731:u32, "FrameThickness(1)"=w730:u32, "HeaderIcon"=w732:u8[][], "BodyBkColor"=w733:u32, "error out"=w750:errorcluster)  [unwired: 5 in, 8 out]
            n315 = call <resource>:"GDSLvIcon_AnalyseViIcon.vi"("ViRef/LvCLassRef/LvLibRef/ViPath"=w734, "error in (no error)"=w750) -> ("BodyIcon"=w737:u8[][], "BodyBkColor"=w735:u32, "error out"=w736:errorcluster)  [unwired: 5 in, 10 out]
            n316 = call <resource>:"GDSLvIcon_ReplaceIconColor.vi"("IconIn"=w737, "OldColor"=w735, "NewColor"=w733, "error in (no error)"=w736) -> ("IconOut"=w745:u8[][], "error out"=w743:errorcluster)  [unwired: 14 in]
            n317 = call <resource>:"GDSLvIcon_CreateIconPicture.vi"("FrameColor"=w731, "FrameThickness(1)"=w730, "HeaderIconIn"=w732, "BodyIconIn"=w745, "error in (no error)"=w743) -> ("WholeIconOut"=w740:u8[][], "error out"=w744:errorcluster)  [unwired: 9 in, 4 out]
            n318 = Reshape Array(w740, 1024 ("dimension size")) -> (w742:u8[])
            n319 = Bundle By Name(cluster=T7 {"image type"=0, "image depth"=8, "image"=[], "mask"=[], "colors"=[], "Rectangle"={"left"=0, "top"=0, "right"=32, "bottom"=32}} ("image data"), "image"=w742) -> (w739:T7)
            n320 = invoke class="VI" method="VI Icon.Set from Image Data"(reference=w734, error in=w744, "ImageData"=w739) -> (reference out=w747:refnum<vi>, error out=w746:errorcluster)  [unwired: 3 in, 4 out]
            n321 = call <resource>:"Scripting_SaveVi.vi"("ForceResaving(False)"=TRUE, "error in (no error)"=w746, "VIRefToSaveIn"=w747) -> ("error out"=w728:errorcluster)  [unwired: 7 in, 1 out]
            n322 = Close Reference(reference=w729, error in (no error)=w728) -> ()  [unwired: 1 out]
          }
          frame "AddImplementVIInInterfaceSubClass" {
            w778 = refnum<vi> refnum  # NamedBundler
            n323 = Unbundle By Name(w764) -> ("RefNameInSubInterface"=w765:string, "NewInterfaceClassRef"=w767:refnum<vi>)
            n324 = Unbundle By Name(w764) -> ("Application"=w798:refnum<vi>, "ImplementVI"=w804:path, "ClassName"=w800:string)
            n325 = property class="LVClassLibrary"(reference=w767) -> (reference out=w785:refnum<vi>, "Path"=w803:path)  [unwired: 1 in, 1 out]
            n326 = call <resource>:"GDSLvClass_GetClassInfo.vi"("Class Refnum In"=w766, "error in (no error)"=w791) -> ("ClassMemberPath"=w789:path, "error out"=w790:errorcluster)  [unwired: 14 in, 2 out]
            n327 = Strip Path(path=w803) -> (stripped path=w799:path)  [unwired: 1 out]
            n328 = Format Into String(format string="%s_Implement.vi", w800) -> (resulting string=w801:string)  [unwired: 2 in, 1 out]
            n329 = call <resource>:"GDSLvClass_GetClassInfo.vi"("Class Refnum In"=w785, "error in (no error)"=w790) -> ("Class Refnum Out"=w784:refnum<vi>, "ClassMemberPath"=w788:path, "error out"=w792:errorcluster)  [unwired: 14 in, 1 out]
            n330 = Build Path(base path=w799, name or relative path=w801) -> (appended path=w759:path)
            n331 = Copy(8:w792, 10:w759, 11:w804) -> (0:w760:errorcluster)  [unwired: 2 in, 2 out]
            n332 = Set Permissions(7:i16 511 ("permissions"), 8:w760, 11:w759) -> (0:w757:errorcluster, 3:w758:path)  [unwired: 2 in]
            n333 = Open VI Reference(application reference (local)=w798, vi path=w758, error in (no error)=w757) -> (vi reference=w762:refnum<vi>, error out=w796:errorcluster)  [unwired: 3 in]
            n334 = Build Array(w765) -> (w773:string[])
            n335 = Bundle(w773) -> (w772:cluster{string[]})  [unwired: 1 in]
            n336 = property class="VI"(reference=w762, error in=w796) -> (reference out=w787:refnum<vi>, error out=w782:errorcluster, "Panel"=w797:refnum<vi>)
            n337 = Bundle By Name(cluster=w764, "SubInterfaceImplementVI"=w759, "ImplementViRef"=w762) -> (w763:T3)
            n338 = Build Array(w772) -> (w771:cluster{string[]}[])
            n339 = property class="Pnl"(reference=w797, error in=w782) -> (reference out=w783:refnum<vi>, error out=w794:errorcluster, "Controls[]"=w795:refnum<vi>[])
            n340 = for {
              tunnel: w795 -> [w813] mode=indexing
              shift-right: [w808] -> w793
              shift-left: w794 -> [w810]
              tunnel: w789 -> [w806]
              tunnel: w788 -> [w805]
              n341 = property class="Ctl"(reference=w813, error in=w810) -> (reference out=w807:refnum<vi>, error out=w809:errorcluster, "Label.Text"=w812:string, "ClassName"=w811:string)
              n342 = case shown="\"LabVIEWClassControl\"" w811 {
                tunnel: w812 -> [_ w825]
                tunnel: [w815 w819] -> w808
                tunnel: w809 -> [w815 w820]
                tunnel: w807 -> [w814 w822]
                tunnel: w806 -> [_ w817]
                tunnel: w805 -> [_ w816]
                frame "False", Default {
                  n343 = Close Reference(reference=w814) -> ()  [unwired: 1 in, 1 out]
                }
                frame "LabVIEWClassControl" {
                  n344 = Equal?(x=w825, y="ClassThatImplements") -> (x = y?=w823:bool)
                  n345 = Select(t=w817, s=w823, f=w816) -> (s? t:f=w818:path)
                  n346 = invoke class="Ctl" method="Replace"(reference=w822, error in=w820, "Path"=w818) -> (reference out=w821:refnum<vi>, error out=w819:errorcluster)  [unwired: 3 in, 4 out]
                  n347 = Close Reference(reference=w821) -> ()  [unwired: 1 in, 1 out]
                }
              }
            }
            n348 = Close Reference(reference=w783, error in (no error)=w793) -> (error out=w769:errorcluster)
            n349 = call <resource>:"Scripting_FindNodeOnDiagram.vi"("ViRef(Ignored If Not Wired)"=w762, "NodeTypesToSearchFor"=string[] ["NamedBundler"], "error in (no error)"=w769) -> ("Nodes"=w774:refnum<vi>[], "error out"=w779:errorcluster)  [unwired: 15 in]
            n350 = Index Array(array=w774) -> (element=w780:refnum<vi>)  [unwired: 1 in]
            n351 = To More Specific Class(target class=w778, reference=w780, error in=w779) -> (specific class reference=w777:refnum<vi>, error out=w776:errorcluster)
            n352 = property class="NmdBndl"(reference=w777, error in=w776, "FullElemNms[]"=w771) -> (error out=w775:errorcluster)  [unwired: 1 out]
            n353 = Close Reference(reference=w774, error in (no error)=w775) -> (error out=w770:errorcluster)
            n354 = invoke class="LVClassLibrary" method="AddFile"(reference=w784, error in=w770, "Path"=w759) -> (error out=w756:errorcluster)  [unwired: 1 in, 3 out]
            n355 = call <resource>:"CommonVIs_Wait.vi"("error in"=w756) -> ("error out"=w755:errorcluster)  [unwired: 9 in]
            n356 = invoke class="VI" method="Save.Instrument"(reference=w787, error in=w755) -> (error out=w786:errorcluster)  [unwired: 4 in, 5 out]
          }
          frame "UpdateImplementIcon" {
            n357 = Unbundle By Name(w853) -> ("ImplementViRef"=w835:refnum<vi>, "NewInterfaceClassRef"=w828:refnum<vi>)
            n358 = property class="LVClassLibrary" props=["Path", "Member Data"](reference=w828, error in=w852) -> (error out=w850:errorcluster, "Member Data"=w827:refnum<vi>)  [unwired: 2 out]
            n359 = call <resource>:"GDSLvIcon_AnalyseViIcon.vi"("ViRef/LvCLassRef/LvLibRef/ViPath"=w827, "error in (no error)"=w850) -> ("FrameColor"=w832:u32, "FrameThickness(1)"=w831:u32, "HeaderIcon"=w833:u8[][], "BodyBkColor"=w834:u32, "error out"=w851:errorcluster)  [unwired: 5 in, 8 out]
            n360 = call <resource>:"GDSLvIcon_AnalyseViIcon.vi"("ViRef/LvCLassRef/LvLibRef/ViPath"=w835, "error in (no error)"=w851) -> ("BodyIcon"=w838:u8[][], "BodyBkColor"=w836:u32, "error out"=w837:errorcluster)  [unwired: 5 in, 10 out]
            n361 = call <resource>:"GDSLvIcon_ReplaceIconColor.vi"("IconIn"=w838, "OldColor"=w836, "NewColor"=w834, "error in (no error)"=w837) -> ("IconOut"=w846:u8[][], "error out"=w844:errorcluster)  [unwired: 14 in]
            n362 = call <resource>:"GDSLvIcon_CreateIconPicture.vi"("FrameColor"=w832, "FrameThickness(1)"=w831, "HeaderIconIn"=w833, "BodyIconIn"=w846, "error in (no error)"=w844, "ImageRows(32)"=17) -> ("WholeIconOut"=w841:u8[][], "error out"=w845:errorcluster)  [unwired: 8 in, 4 out]
            n363 = Reshape Array(w841, 1024 ("dimension size")) -> (w843:u8[])
            n364 = Bundle By Name(cluster=T7 {"image type"=0, "image depth"=8, "image"=[], "mask"=[], "colors"=[], "Rectangle"={"left"=0, "top"=0, "right"=32, "bottom"=32}} ("image data"), "image"=w843) -> (w840:T7)
            n365 = invoke class="VI" method="VI Icon.Set from Image Data"(reference=w835, error in=w845, "ImageData"=w840) -> (reference out=w848:refnum<vi>, error out=w847:errorcluster)  [unwired: 3 in, 4 out]
            n366 = call <resource>:"Scripting_SaveVi.vi"("ForceResaving(False)"=TRUE, "error in (no error)"=w847, "VIRefToSaveIn"=w848) -> ("error out"=w826:errorcluster)  [unwired: 7 in, 1 out]
            n367 = Close Reference(reference=w827, error in (no error)=w826) -> ()  [unwired: 1 out]
          }
          frame "UpdateConstructor" {
            n368 = Unbundle By Name(w860) -> ("Application"=w859:refnum<vi>, "SubInterfaceImplementVI"=w858:path, "RefNameInClass"=w857:string)
            n369 = call <resource>:"Interface_AddImplementVI.vi"("Application"=w859, "ClassRefToActOn"=w854, "RefNameInClass"=w857, "SubInterfaceImplementVI"=w858, "error in"=w856) -> ("error out"=w855:errorcluster)  [unwired: 14 in]
          }
          frame "CloseDown", "CloseRefs", "Error", Default {
            n370 = Unbundle By Name(w865) -> ("BaseInterfaceClassRef"=w873:refnum<vi>, "NewInterfaceClassRef"=w863:refnum<vi>, "C_MethodRefs"=w876:refnum<vi>[], "I_MethodRefs"=w875:refnum<vi>[], "Application"=w874:refnum<vi>, "GetVIRef"=w868:refnum<vi>, "ImplementViRef"=w867:refnum<vi>)
            n371 = call <resource>:"GDSError_LogErrorInformation.vi"("State"=w866, "LocalVariableData"=w865, "error in (no error)"=w864) -> ()  [unwired: 16 in, 1 out]
            n372 = call <resource>:"GDSLvClass_SaveEverythingInClass.vi"("ClassRefIn"=w871, "ForceResaving(False)"=TRUE, "error in"=w864) -> ("error out"=w870:errorcluster)  [unwired: 15 in, 1 out]
            n373 = Not A Number/Path/Refnum?(number/path/refnum=w863) -> (NaN/Path/Refnum?=w862:bool)
            n374 = case shown="True" w862 {
              tunnel: w870 -> [w880 w882]
              tunnel: w863 -> [w879 _]
              tunnel: [w878 w882] -> w869
              frame False {
                n375 = call <resource>:"GDSLvClass_SaveEverythingInClass.vi"("ClassRefIn"=w879, "ForceResaving(False)"=TRUE, "error in"=w880) -> ("error out"=w878:errorcluster)  [unwired: 15 in, 1 out]
              }
              frame True {
              }
            }
            n376 = stacked-sequence {
              tunnel: w876 -> [w889]
              tunnel: w875 -> [w888]
              tunnel: w874 -> [w887]
              tunnel: w863 -> [w886]
              tunnel: w873 -> [w885]
              tunnel: w869 -> [_]
              tunnel: w868 -> [w884]
              tunnel: w867 -> [w883]
              frame #0 {
                n377 = Close Reference(reference=w889) -> ()  [unwired: 1 in, 1 out]
                n378 = Close Reference(reference=w888) -> ()  [unwired: 1 in, 1 out]
                n379 = Close Reference(reference=w887) -> ()  [unwired: 1 in, 1 out]
                n380 = Close Reference(reference=w884) -> ()  [unwired: 1 in, 1 out]
                n381 = Close Reference(reference=w883) -> ()  [unwired: 1 in, 1 out]
                n382 = Close Reference(reference=w885) -> ()  [unwired: 1 in, 1 out]
                n383 = Close Reference(reference=w886) -> ()  [unwired: 1 in, 1 out]
              }
            }
          }
        }
        n384 = Equal?(x=w145, y="Exit") -> (x = y?=w148:bool)
        n385 = Select(t="Error", s=w144, f=w145) -> (s? t:f=w149:string)
      }
    }
    frame "CreatePatternMethod" {
      n386 = property class="VI"(error in=w891, "Front Panel.Open"=FALSE ("Front Panel Window:Open")) -> (error out=w890:errorcluster)  [unwired: 1 in, 1 out]
    }
  }
  "error out" <- w8
  "DataOut" <- w5
  "Cancelled" <- w6
  "Name" <- "Interface" ("Name")
